vi "MultiPAS-IV.vi"() -> ()   [LabVIEW 2011]
uses:
  Desktop/__fcncfs4.franklin.uga.edu_CHEM/Groups/Smith_G/Photoacoutic Spectroscopy/PAS-CRD/Get Tau/Analysis/analys_meth.ctl
  <vilib>/Analysis/4window.llb/windowTd.ctl
  sub/QMH/QMH Add Message to Queue (Single Element).vi
  sub/QMH/QMH Add Message to Queue (Array).vi
  <vilib>/measure/maspectr.llb/FFT Spectrum (Mag-Phase) for 1 Chan.vi
  sub/fftGetMags_IV.vi
  sub/rollingAverage_IV.vi
  sub/micUnbundle_IV.vi
  sub/laserDiagnose_IV.vi
  <vilib>/Instr/_visa.llb/VISA Configure Serial Port (Instr).vi
  sub/lasersSetFrequencies_IV.vi
  sub/absCalcPlot_IV.vi
  sub/pdNormalize_IV.vi
  <vilib>/measure/NI_MAPro.lvlib
  <vilib>/Analysis/NI_AALPro.lvlib
panel:
  out "Channel A":cluster{i32, sgl, "Data (mV)":dbl[]}(graph)
  out "tau":dbl(graph)
  in  "785 Emission":bool
  in  "785 Power (mW)":dbl(slide)=100.0 min=0.0 max=100.0 step=1.0 scale=0.0..100.0
  out "PAS Save":bool caption="Overtemp"
  in  "Data 2":i32[][](array[numeric])=[[-16374, -7248, 2543, 12030, 20279, 26487, 30037, 30583, 28073, 22744, 15131, 5976, -3818, -13288, -21504, -27663, -31155, -31636, -29064, -23686, -16036, -6862, 2936, 12388, 20571, 26684, 30122, 30546, 27911, 22483, 14793, 5595, -4207, -13644, -21795, -27855, -31232, -31591, -28898, -23423, -15695, -6476, 3323, 12743, 20858, 26873, 30194, 30492, 27744, 22213, 14447, 5207, -4597, -14002, -22082, -28044, -31304, -31540, -28731, -23149, -15348, -6093, 3713, 13101, 21145, 27063, 30265, 30442, 27576, 21943, 14103, 4822, -4984, -14354, -22365, -28230, -31373, -31485, -28556, -22876, -14998, -5702, 4104, 13452, 21428, 27245, 30335, 30388, 27400, 21669, 13754, 4435, -5375, -14705, -22643, -28407, -31436, -31426, -28378, -22598, -14648, -5314, 4497, 13803, 21706, 27423, 30394, 30325, 27221, 21390, 13402, 4045, -5763, -15056, -22921, -28586, -31496, -31361, -28198, -22319, -14297, -4924, 4879, 14151, 21982, 27597, 30451, 30257, 27038, 21107, 13050, 3658, -6149, -15402, -23193, -28754, -31546, -31290, -28010, -22033, -13944, -4536, 5266, 14498, 22252, 27767, 30500, 30184, 26849, 20821, 12696, 3267, -6535, -15748, -23462, -28924, -31596, -31216, -27821, -21748, -13587, -4147, 5653, 14838, 22519, 27930, 30549, 30110, 26658, 20535, 12337, 2878, -6919, -16089, -23727, -29087, -31641, -31137, -27627, -21457, -13229, -3753, 6038, 15181, 22786, 28093, 30591, 30031, 26461, 20243, 11979, 2485, -7303, -16428, -23991, -29244, -31678, -31053, -27426, -21159, -12867, -3360, 6424, 15524, 23043, 28252, 30633, 29946, 26262, 19946, 11617, 2096, -7686, -16764, -24246, -29398, -31712, -30964, -27224, -20862, -12503, -2971, 6803, 15859, 23301, 28401, 30661, 29852, 26058, 19648, 11254, 1703, -8069, -17099, -24500, -29547, -31741, -30870, -27018, -20562, -12138, -2575, 7188, 16192, 23556, 28549, 30689, 29756, 25848, 19348, 10891, 1312, -8448, -17430, -24753, -29691, -31765, -30773, -26806, -20259, -11775, -2186, 7566, 16521, 23801, 28690, 30709, 29656, 25634, 19038, 10523, 919, -8831, -17762, -24997, -29833, -31788, -30672, -26593, -19955, -11409, -1792, 7944, 16850, 24047, 28830, 30724, 29548, 25416, 18729, 10152, 523, -9212, -18092, -25245, -29969, -31805, -30566, -26375, -19647, -11041, -1403, 8319, 17173, 24287, 28963, 30734, 29436, 25192, 18418, 9781, 130, -9587, -18413, -25481, -30101, -31814, -30449, -26150, -19332, -10666, -1007, 8697, 17497, 24524, 29090, 30745, 29325, 24968, 18105, 9408, -263, -9962, -18735, -25718, -30228, -31820, -30334, -25921, -19016, -10296, -618, 9072, 17814, 24756, 29213, 30746, 29202, 24738, 17787, 9036, -657, -10338, -19058, -25951, -30350, -31818, -30214, -25690, -18699, -9922, -224, 9442, 18128, 24984, 29330, 30738, 29078, 24502, 17466, 8658, -1050, -10710, -19371, -26178, -30467, -31814, -30088, -25458, -18382, -9550, 167, 9812, 18440, 25206, 29443, 30732, 28947, 24264, 17143, 8281, -1445, -11083, -19685, -26404, -30581, -31807, -29959, -25221, -18059, -9175, 556, 10178, 18750, 25426, 29548, 30718, 28809, 24018, 16812, 7901, -1842, -11457, -19996, -26624, -30690, -31795, -29824, -24980, -17733, -8799, 950, 10549, 19058, 25643, 29655, 30700, 28673, 23773, 16484, 7523, -2235, -11824, -20304, -26840, -30793, -31772, -29682, -24731, -17402, -8415, 1341, 10916, 19363, 25856, 29755, 30677, 28528, 23522, 16151, 7141, -2626, -12191, -20607, -27051, -30891, -31746, -29536, -24481, -17070, -8035, 1733, 11280, 19664, 26064, 29851, 30648, 28381, 23272, 15818, 6762, -3019, -12555, -20906, -27258, -30984, -31717, -29391, -24226, -16736, -7655, 2128, 11641, 19962, 26270, 29940, 30615, 28229, 23013, 15483, 6376, -3409, -12914, -21204, -27459, -31071, -31684, -29236, -23967, -16398, -7271, 2515, 12005, 20258, 26468, 30024, 30577, 28072, 22753, 15143, 5990, -3802, -13276, -21497, -27660, -31157, -31643, -29076, -23707, -16058, -6886, 2908, 12363, 20550, 26666, 30107, 30536, 27914, 22489, 14805, 5607, -4192, -13633, -21787, -27849, -31230, -31597, -28911, -23438, -15716, -6501, 3298, 12719, 20839, 26858, 30182, 30488, 27744, 22223, 14459, 5225, -4579, -13988, -22071, -28040, -31304, -31549, -28743, -23167, -15368, -6113, 3693, 13076, 21126, 27047, 30255, 30438, 27576, 21950, 14113, 4837, -4971, -14340, -22354, -28224, -31375, -31494, -28570, -22895, -15022, -5725, 4080, 13430, 21408, 27230, 30324, 30384, 27402, 21676, 13766, 4449, -5360, -14694, -22636, -28409, -31440, -31436, -28397, -22617, -14674, -5338, 4467, 13781, 21686, 27408, 30385, 30320, 27224, 21398, 13418, 4062, -5748, -15044, -22913, -28584, -31498, -31368, -28212, -22339, -14321, -4948, 4856, 14131, 21963, 27583, 30440, 30254, 27042, 21118, 13062, 3669, -6137, -15390, -23183, -28751, -31551, -31297, -28024, -22049, -13962, -4556, 5245, 14476, 22235, 27754, 30497, 30186, 26857, 20834, 12710, 3283, -6519, -15733, -23453, -28921, -31600, -31226, -27837, -21765, -13610, -4168, 5628, 14820, 22502, 27918, 30540, 30109, 26664, 20544, 12354, 2891, -6906, -16074, -23719, -29085, -31646, -31148, -27642, -21475, -13251, -3777, 6014, 15160, 22765, 28078, 30583, 30027, 26468, 20251, 11994, 2501, -7292, -16415, -23980, -29242, -31682, -31064, -27443, -21181, -12892, -3386, 6397, 15501, 23026, 28238, 30624, 29944, 26269, 19959, 11633, 2110, -7673, -16753, -24239, -29395, -31719, -30974, -27239, -20882, -12528, -2993, 6782, 15835, 23285, 28390, 30651, 29852, 26063, 19660, 11271, 1720, -8053, -17087, -24493, -29546, -31746, -30880, -27031, -20583, -12163, -2599, 7166, 16173, 23538, 28538, 30684, 29758, 25853, 19356, 10906, 1327, -8433, -17416, -24743, -29688, -31769, -30782, -26821, -20280, -11797, -2208, 7543, 16501, 23786, 28680, 30704, 29656, 25642, 19053, 10540, 936, -8814, -17747, -24989, -29827, -31787, -30678, -26606, -19973, -11430, -1817, 7923, 16829, 24031, 28819, 30721, 29552, 25424, 18746, 10174, 543, -9191, -18072, -25231, -29962, -31802, -30567, -26384, -19660, -11057, -1422, 8302, 17159, 24274, 28952, 30738, 29443, 25205, 18435, 9801, 150, -9568, -18401, -25472, -30095, -31811, -30457, -26163, -19349, -10687, -1031, 8679, 17481, 24511, 29082, 30742, 29327, 24979, 18121, 9431, -241, -9943, -18717, -25707, -30221, -31815, -30337, -25930, -19029, -10312, -631, 9058, 17802, 24745, 29207, 30746, 29209, 24750, 17805, 9057, -634, -10316, -19037, -25937, -30340, -31814, -30217, -25700, -18713, -9939, -240, 9429, 18117, 24976, 29328, 30740, 29088, 24519, 17486, 8682, -1027, -10688, -19352, -26164, -30458, -31810, -30091, -25465, -18390, -9561, 154, 9800, 18433, 25201, 29442, 30735, 28959, 24282, 17165, 8308, -1420, -11063, -19665, -26386, -30570, -31801, -29961, -25227, -18068, -9185, 547, 10171, 18745, 25424, 29552, 30726, 28825, 24038, 16835, 7925, -1815, -11429, -19974, -26608, -30681, -31789, -29826, -24984, -17741, -8807, 938, 10536, 19047, 25636, 29657, 30708, 28685, 23794, 16510, 7550, -2205, -11798, -20280, -26821, -30782, -31766, -29684, -24737, -17411, -8429, 1331, 10906, 19356, 25851, 29758, 30684, 28544, 23546, 16178, 7169, -2598, -12162, -20582, -27035, -30879, -31744, -29540, -24485, -17080, -8048, 1721, 11267, 19655, 26061, 29852, 30654, 28395, 23291, 15843, 6786, -2993, -12527, -20884, -27240, -30974, -31713, -29390, -24230, -16744, -7662, 2115, 11635, 19957, 26268, 29945, 30624, 28246, 23035, 15509, 6406, -3382, -12889, -21180, -27444, -31061, -31677, -29236, -23975, -16408, -7284], [-19329, -1252, 17344, 29341, 30145, 19451, 1353, -17227, -29174, -29920, -19175, -1056, 17506, 29408, 30095, 19300, 1159, -17387, -29238, -29860, -19019, -860, 17671, 29475, 30037, 19143, 960, -17553, -29307, -29809, -18866, -664, 17832, 29545, 29987, 18991, 771, -17707, -29365, -29749, -18707, -466, 17992, 29605, 29926, 18832, 570, -17873, -29434, -29694, -18556, -272, 18151, 29670, 29869, 18676, 375, -18031, -29495, -29633, -18395, -75, 18310, 29729, 29809, 18516, 175, -18194, -29561, -29579, -18238, 120, 18469, 29792, 29750, 18362, -17, -18347, -29617, -29515, -18076, 316, 18629, 29848, 29682, 18197, -218, -18510, -29679, -29456, -17921, 513, 18787, 29910, 29626, 18042, -408, -18664, -29734, -29388, -17757, 709, 18941, 29965, 29560, 17875, -609, -18823, -29791, -29326, -17600, 904, 19095, 30023, 29495, 17717, -802, -18975, -29845, -29260, -17434, 1099, 19251, 30075, 29425, 17551, -1001, -19131, -29901, -29194, -17277, 1296, 19408, 30130, 29359, 17393, -1193, -19284, -29953, -29124, -17112, 1491, 19560, 30184, 29290, 17225, -1392, -19440, -30008, -29056, -16949, 1686, 19713, 30237, 29226, 17069, -1581, -19587, -30054, -28982, -16781, 1883, 19866, 30287, 29151, 16898, -1781, -19742, -30107, -28913, -16616, 2079, 20018, 30337, 29082, 16737, -1973, -19888, -30152, -28838, -16449, 2275, 20167, 30383, 29006, 16564, -2174, -20041, -30200, -28765, -16282, 2471, 20321, 30430, 28934, 16403, -2364, -20187, -30243, -28688, -16113, 2669, 20465, 30470, 28853, 16230, -2568, -20341, -30294, -28618, -15953, 2860, 20615, 30519, 28783, 16070, -2755, -20486, -30335, -28537, -15779, 3057, 20760, 30560, 28700, 15892, -2956, -20637, -30378, -28461, -15613, 3252, 20909, 30605, 28628, 15730, -3145, -20777, -30418, -28377, -15440, 3446, 21054, 30645, 28543, 15557, -3345, -20927, -30460, -28299, -15271, 3643, 21199, 30686, 28465, 15391, -3534, -21066, -30495, -28215, -15100, 3839, 21345, 30722, 28380, 15214, -3734, -21213, -30534, -28134, -14928, 4032, 21487, 30760, 28300, 15044, -3926, -21355, -30570, -28052, -14757, 4225, 21627, 30792, 28209, 14870, -4123, -21501, -30607, -27968, -14586, 4419, 21768, 30832, 28129, 14702, -4314, -21637, -30639, -27880, -14413, 4612, 21907, 30859, 28040, 14521, -4515, -21780, -30675, -27796, -14241, 4804, 22048, 30895, 27953, 14352, -4702, -21919, -30705, -27707, -14064, 4999, 22187, 30922, 27859, 14172, -4900, -22060, -30739, -27620, -13892, 5193, 22326, 30954, 27773, 14003, -5090, -22194, -30765, -27524, -13712, 5386, 22462, 30981, 27679, 13823, -5285, -22333, -30794, -27436, -13538, 5580, 22600, 31013, 27591, 13650, -5476, -22466, -30820, -27343, -13363, 5770, 22732, 31033, 27491, 13468, -5673, -22605, -30848, -27251, -13187, 5964, 22870, 31060, 27401, 13292, -5863, -22736, -30870, -27155, -13010, 6156, 23000, 31079, 27299, 13111, -6058, -22873, -30895, -27060, -12833, 6347, 23134, 31104, 27208, 12936, -6248, -23004, -30918, -26965, -12652, 6536, 23260, 31120, 27106, 12753, -6444, -23136, -30939, -26865, -12472, 6729, 23395, 31148, 27011, 12578, -6634, -23266, -30959, -26766, -12296, 6919, 23523, 31161, 26907, 12392, -6830, -23402, -30982, -26665, -12115, 7109, 23652, 31180, 26809, 12213, -7016, -23524, -30992, -26564, -11932, 7301, 23777, 31195, 26704, 12032, -7210, -23655, -31011, -26464, -11755, 7492, 23907, 31211, 26605, 11855, -7395, -23778, -31024, -26358, -11573, 7680, 24031, 31218, 26494, 11665, -7592, -23908, -31039, -26258, -11392, 7871, 24158, 31237, 26394, 11491, -7775, -24031, -31050, -26153, -11210, 8063, 24281, 31247, 26285, 11302, -7972, -24159, -31062, -26046, -11027, 8250, 24407, 31258, 26180, 11124, -8157, -24276, -31067, -25937, -10841, 8438, 24526, 31265, 26071, 10936, -8347, -24401, -31078, -25829, -10659, 8630, 24649, 31275, 25965, 10755, -8533, -24522, -31087, -25721, -10474, 8816, 24770, 31280, 25853, 10566, -8726, -24641, -31091, -25608, -10290, 9003, 24891, 31287, 25746, 10386, -8910, -24756, -31095, -25498, -10105, 9192, 25008, 31287, 25627, 10196, -9102, -24881, -31101, -25386, -9919, 9381, 25127, 31296, 25521, 10019, -9284, -24994, -31099, -25268, -9732, 9570, 25243, 31293, 25403, 9826, -9476, -25113, -31105, -25157, -9544, 9756, 25359, 31298, 25291, 9645, -9655, -25225, -31099, -25040, -9359, 9942, 25473, 31291, 25167, 9453, -9847, -25341, -31102, -24926, -9173, 10124, 25586, 31294, 25057, 9269, -10029, -25450, -31095, -24809, -8986, 10310, 25696, 31284, 24931, 9078, -10218, -25564, -31094, -24688, -8798, 10497, 25812, 31287, 24819, 8896, -10399, -25673, -31085, -24567, -8608, 10682, 25922, 31278, 24698, 8703, -10587, -25785, -31080, -24448, -8422, 10866, 26033, 31274, 24582, 8522, -10765, -25890, -31067, -24321, -8230, 11050, 26140, 31263, 24455, 8325, -10952, -26001, -31064, -24201, -8040, 11234, 26248, 31255, 24338, 8142, -11132, -26106, -31054, -24079, -7852, 11417, 26353, 31243, 24207, 7948, -11316, -26217, -31041, -23952, -7662, 11601, 26464, 31236, 24089, 7763, -11494, -26315, -31025, -23829, -7471, 11782, 26562, 31217, 23957, 7567, -11682, -26422, -31014, -23702, -7282, 11962, 26667, 31205, 23834, 7383, -11859, -26521, -30998, -23575, -7092, 12144, 26770, 31187, 23704, 7186, -12043, -26626, -30981, -23444, -6900, 12328, 26875, 31176, 23582, 7003, -12218, -26724, -30962, -23316, -6709, 12505, 26971, 31154, 23446, 6805, -12401, -26825, -30946, -23189, -6517, 12687, 27073, 31139, 23322, 6620, -12576, -26919, -30922, -23054, -6323, 12867, 27170, 31114, 23185, 6422, -12760, -27022, -30904, -22923, -6132, 13047, 27272, 31096, 23060, 6237, -12934, -27114, -30879, -22790, -5940, 13222, 27362, 31068, 22921, 6041, -13116, -27212, -30855, -22657, -5748, 13401, 27461, 31048, 22790, 5853, -13289, -27302, -30828, -22522, -5555, 13577, 27549, 31019, 22652, 5652, -13472, -27398, -30806, -22388, -5362, 13753, 27645, 30995, 22521, 5463, -13642, -27487, -30776, -22248, -5169, 13928, 27733, 30963, 22376, 5266, -13823, -27584, -30750, -22113, -4975, 14106, 27828, 30937, 22246, 5082, -13992, -27669, -30717, -21974, -4782, 14280, 27914, 30902, 22101, 4880, -14174, -27760, -30689, -21837, -4588, 14454, 28006, 30875, 21965, 4692, -14340, -27843, -30653, -21693, -4391, 14631, 28092, 30840, 21822, 4494, -14519, -27934, -30620, -21552, -4198, 14805, 28179, 30808, 21688, 4308, -14687, -28015, -30582, -21410, -4004, 14975, 28262, 30770, 21540, 4106, -14861, -28103, -30548, -21268, -3808, 15149, 28349, 30739, 21402, 3916, -15032, -28183, -30512, -21124, -3614, 15319, 28430, 30697, 21255, 3715, -15205, -28267, -30475, -20982, -3421, 15490, 28513, 30664, 21116, 3524, -15376, -28348, -30435, -20837, -3225, 15660, 28592, 30617, 20962, 3327, -15550, -28432, -30397, -20695, -3032, 15829, 28673, 30581, 20820, 3134, -15711, -28506, -30353, -20546, -2837, 15994, 28746, 30530, 20669, 2933, -15887, -28585, -30311, -20400, -2641, 16167, 28828, 30496, 20528, 2745, -16052, -28660, -30264, -20248, -2445, 16335, 28901, 30445, 20376, 2544, -16221, -28737, -30219, -20102, -2250, 16505, 28983, 30406, 20231, 2357, -16381, -28808, -30171, -19950, -2053, 16670, 29053, 30355, 20075, 2154, -16552, -28883, -30127, -19803, -1859, 16835, 29128, 30308, 19930, 1965, -16714, -28952, -30073, -19650, -1663, 17001, 29192, 30255, 19772, 1764, -16881, -29028, -30026, -19496, -1467, 17165, 29268, 30208, 19626, 1572, -17043, -29095, -29977, -19346]]
  out "Filtering":bool caption="Time has Elapsed"
  in  "Switch Filter":bool
  in  "Auto Filter":bool
  out "Elapsed Time (min)":dbl caption="Elapsed Time (s)" format="%#.1g"
  in  "Filter Length (min)":dbl=6.0 caption="Time Target (s)"
  in  "Sample Length (min)":dbl=24.0 caption="Time Target (s)" format="%#.1f"
  out "Time has Elapsed":bool
  in  "Time Target (s)":dbl=1.0
  in  "sweep":bool
  in  "All Emit":bool
  in  "Alignment Mode":bool
  in  "662 Emission":bool
  in  "662 Power (mW)":dbl(slide)=100.0 min=0.0 max=100.0 step=1.0 scale=0.0..100.0
  in  "532 Emission":bool
  in  "532 Power (mW)":dbl(slide)=80.0 min=0.0 max=80.0 step=1.0 scale=0.0..80.0
  in  "406 Power (mW)":dbl(slide)=100.0 min=0.0 max=100.0 step=1.0 scale=0.0..100.0
  in  "406 Emission":bool
  out "Overtemp":bool
  in  "Tab Control":T1(tab)=enum."Oscilloscope"
  out "crd":path
  in  "785 Port":refnum<visa-resource-name>="COM81"
  in  "785 PD Cal":dbl=0.039
  out "Error Console":T2
  out "pd":path caption="Photodiode File Path"
  out "mic":path caption="Microphone File Path"
  out "processed":path caption="Processed Data File Path"
  out "sweeps":path caption="Frequency Sweeps File Path"
  out "Laser Temperatures":T3(graph)
  in  "pd id":u32=1
  in  "mic id":u32
  in  "mic cal, scu":dbl=5.41531278804282e-05 format="%#_3e"
  in  "mic cal, scu":dbl=5.59307241877627e-05 format="%#_3e"
  in  "406 Port":refnum<visa-resource-name>="COM80"
  in  "532 Port":refnum<visa-resource-name>="COM79"
  in  "662 Port":refnum<visa-resource-name>="COM62"
  in  "Teensy Port":refnum<visa-resource-name>="COM78"
  in  "Save Data":bool
  in  "405 PD Cal 3":dbl=0.052
  in  "532 PD Cal 3":dbl=0.035
  in  "660 PD Cal 3":dbl=0.038
  in  "Channel A Settings":T4={"Enabled"=TRUE, "Coupling"=0, "Range"=1, "Analogue Offset"=0.0} {"Range" items=["20 mV"=1, "50 mV"=2, "100 mV"=3, "200 mV"=4, "500 mV"=5, "1 V"=6, "2 V"=7, "5 V"=8, "10 V"=9, "20 V"=10]; "Coupling" items=["AC", "DC"]}
  in  "Trigger Settings":T5={"Trigger Enabled"=TRUE, "Trigger Source"=enum."Channel B", "Trigger Threshold (V)"=1.0, "Trigger Direction"=3, "Trigger Delay (samples)"=0, "Auto Trigger Time (ms)"=1000} {"Trigger Direction" items=["Rising"=2, "Falling"=3]}
  in  "Acquisition Settings":T6={"Pre-trigger Samples"=0, "Post-trigger Samples"=10000, "Timebase"=1, "Down Sample Ratio"=10, "Oversample"=1, "Number of Captures"=100, "Down-Sample Mode"=4} {"Down-Sample Mode" items=["None"=0, "Aggregate"=1, "Decimate"=2, "Average"=4]; "Down Sample Ratio" min=1 step=1}
  in  "Channel B Settings":T4={"Enabled"=TRUE, "Coupling"=1, "Range"=8, "Analogue Offset"=0.0} {"Range" items=["20 mV"=1, "50 mV"=2, "100 mV"=3, "200 mV"=4, "500 mV"=5, "1 V"=6, "2 V"=7, "5 V"=8, "10 V"=9, "20 V"=10]; "Coupling" items=["AC", "DC"]}
  in  "785 F (Hz)":i32=1371
  out "freqscan":cluster{i32[], "Best Gaussian Fit":dbl[]}[](graph) caption="Frequency Sweep"
  out "sweep progress":dbl(slide) scale=0.0..1.0
  in  "Autosweep?":bool=TRUE
  in  "set freqs":bool
  out "Calculated Resonance (Hz)":dbl=1370.0
  in  "Data Start Frequency (Hz)":i32=1355
  in  "Data End Frequency (Hz)":i32=1405
  in  "423 F (Hz)":i32=1367
  in  "532 F (Hz)":i32=1373
  in  "662 F (Hz)":i32=1369
  in  "Chart Rolling Average":i32=64
  out "pdwave":waveform(i32)(graph) caption="Photodiode Waveform"
  out "pd ts":cluster{dbl, dbl, dbl, dbl}(graph)
  out "pdfft":cluster{"f0":dbl, "df":dbl, "magnitude":dbl[]}(graph) caption="Photodiode FFT"
  in  "rollavg":i32=16 caption="Dispaly Averaging\n(Transfers to Abs!)"
  out "mic ts":T7(graph)
  out "micfft":cluster{"f0":dbl, "df":dbl, "magnitude":dbl[]}(graph) caption="Photodiode FFT"
  out "micwave":waveform(i32)(graph) caption="Photodiode Waveform"
  out "abs/ext":cluster{dbl, dbl, dbl, dbl, "crd":dbl}(graph)
  in  "getbkg":bool
  out "AAE":dbl(graph)
  in  "Bkg Values (mV)":cluster{dbl, dbl, dbl, dbl}
  out "Absorption Spectrum":cluster{dbl[], "Best Power Fit":dbl[]}[](graph)
  in  "cellcal":dbl=100000.0 caption="Cell Calibration Coefficient (mV/mW)"
  in  "tau0":dbl
  out "Status":string
  in  "Exit":bool
  in  "State Variables":cluster{"CurrentFile":path}
  # "MultiPAS-IV | AeroSmith Labs (2017)"
  # "Laser Control"
  # "Filter Control"
  # "Communications"
  # "Sound Card Parameters"
  # "File paths are populated automatically at <...\\My Documents\\MultiPAS Data\\>.  To save in another location, turn on \"Save Data\" and follow the prompts to choose an alternate working directory."
  # "Photodiode Calibration"
  # "Ringdown Time (us):"
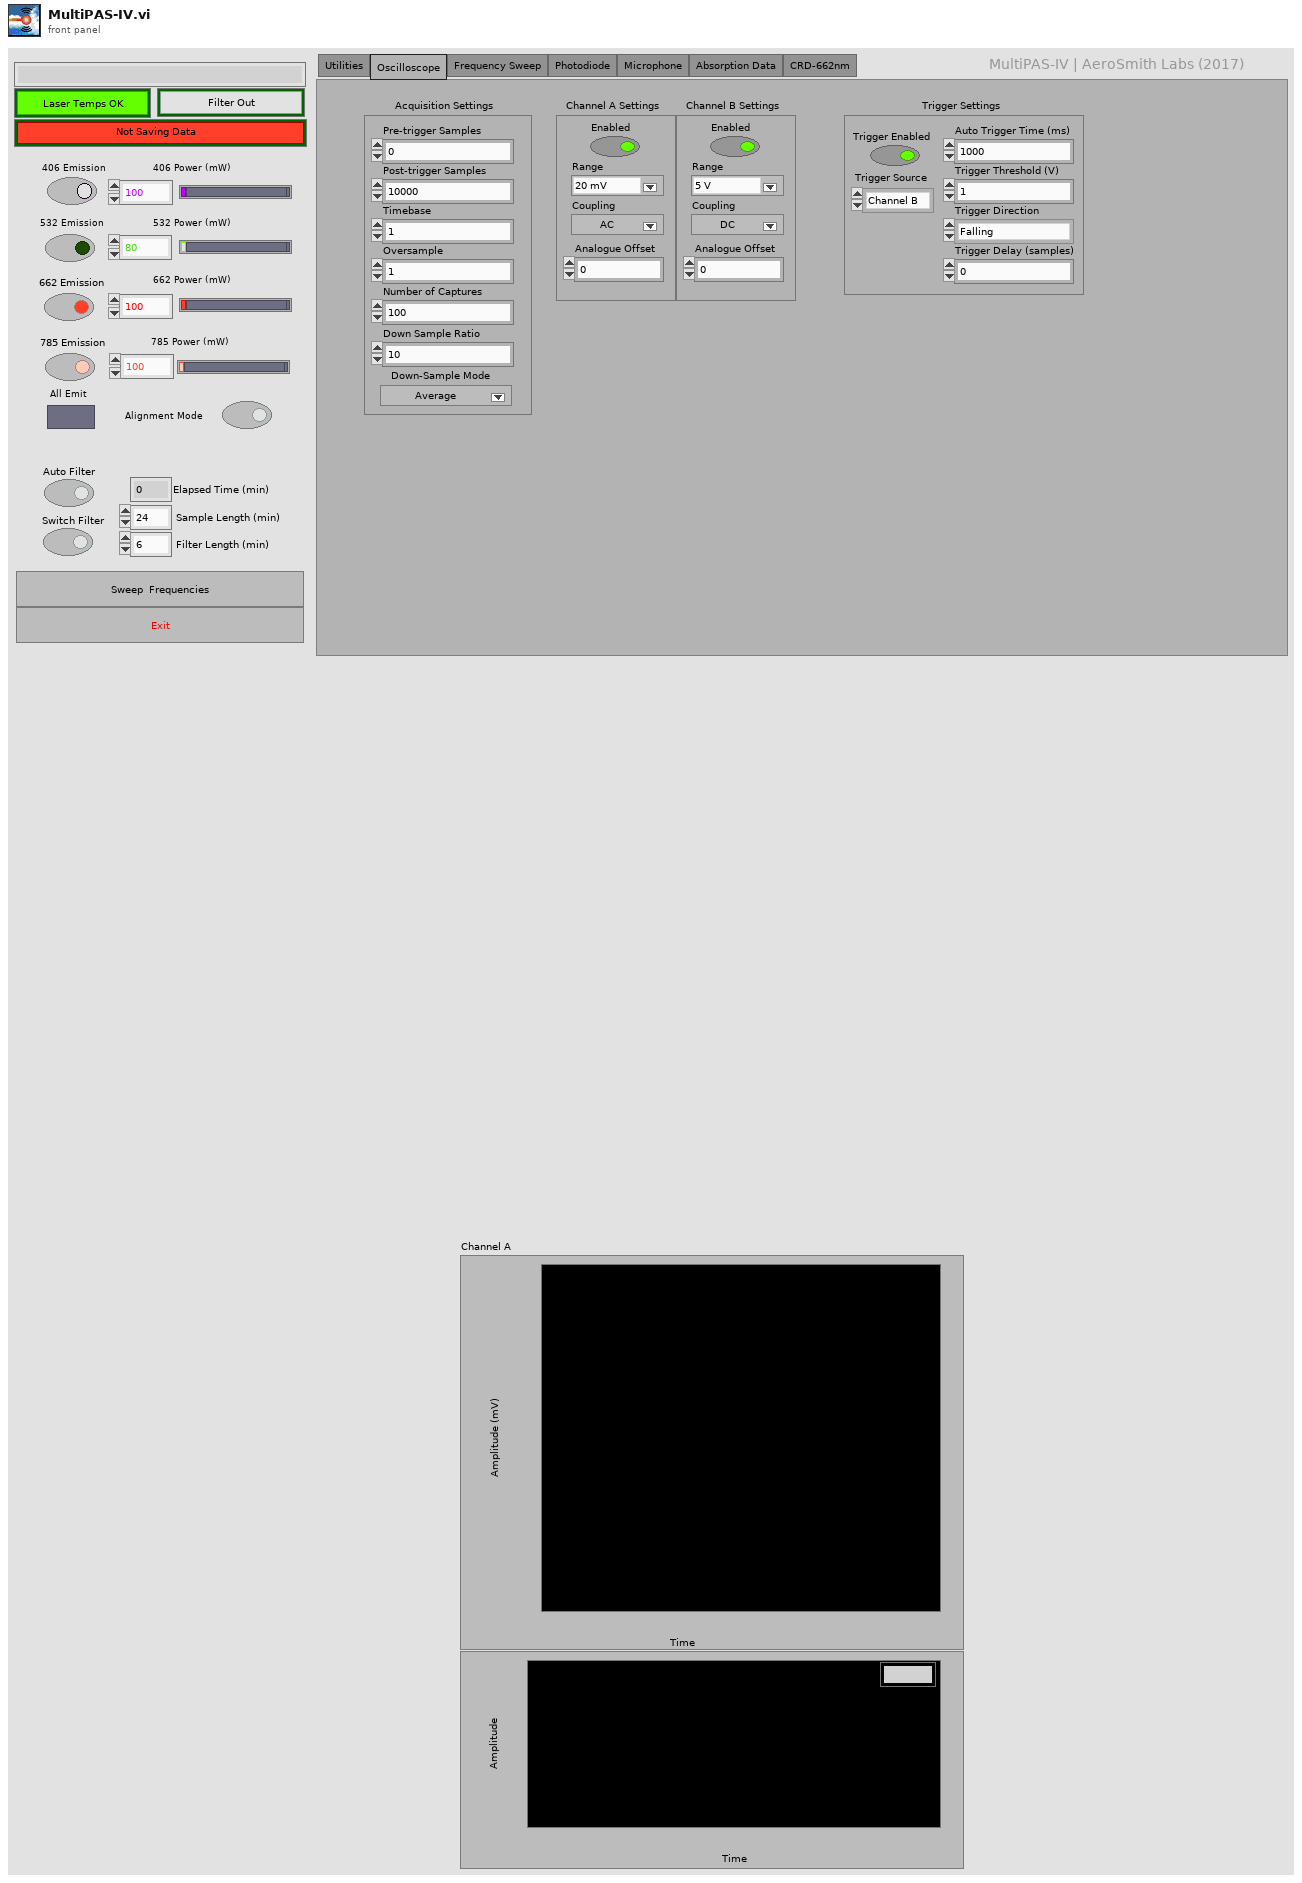
[diagram p1: front panel]
types:
  T1 = enum32{"Utilities", "Oscilloscope", "Frequency Sweep", "Photodiode", "Microphone", "Absorption Data", "CRD-662nm"}
  T2 = cluster{"status":bool, "code":i32, "Message":string}
  T3 = cluster{"Temp (C)":dbl, "Temp (C)":dbl, "Temp (C)":dbl, "Temp (C)":dbl}
  T4 = cluster{"Enabled":bool, "Coupling":i16, "Range":u16, "Analogue Offset":sgl}
  T5 = cluster{"Trigger Enabled":bool, "Trigger Source":enum16{"Channel A", "Channel B", "Channel C", "Channel D", "Ext."}, "Trigger Threshold (V)":dbl, "Trigger Direction":u16, "Trigger Delay (samples)":u32, "Auto Trigger Time (ms)":i16}
  T6 = cluster{"Pre-trigger Samples":u32, "Post-trigger Samples":u32, "Timebase":u32, "Down Sample Ratio":u32, "Oversample":i16, "Number of Captures":u32, "Down-Sample Mode":i32}
  T7 = cluster{"422 Mean":dbl, "532 Mean":dbl, "660 Mean":dbl, "785 Mean":dbl}
  T8 = cluster{"# buffers":i32, "Buffer size":i32, "unit (ms)":enum16{"time (ms)", "Samples"}}
  T9 = typedef "SoundHandle.ctl" = cluster{"DeviceID":u16, "Samples/buf":u32, "Sampl rate":u32, "Bits/sample":u16, "Channels":u8, "Opened":bool}
  T10 = cluster{"405 Mean":dbl, "532 Mean":dbl, "660 Mean":dbl, "660 Mean 2":dbl}
  T11 = typedef "NI_AALPro.lvlib/windowTd.ctl" = u32
  T12 = cluster{"785 New Array":dbl[], "785 Mean":dbl, "785 SD":dbl}
  T13 = cluster{"660 New Array":dbl[], "660 Mean":dbl, "660 SD":dbl}
  T14 = cluster{"532 New Array":dbl[], "532 Mean":dbl, "532 SD":dbl}
  T15 = cluster{"405 New Array":dbl[], "405 Mean":dbl, "405 SD":dbl}
  T16 = typedef "analys_meth.ctl" = enum16{"DFT-1", "DFT-5", "LRS"}
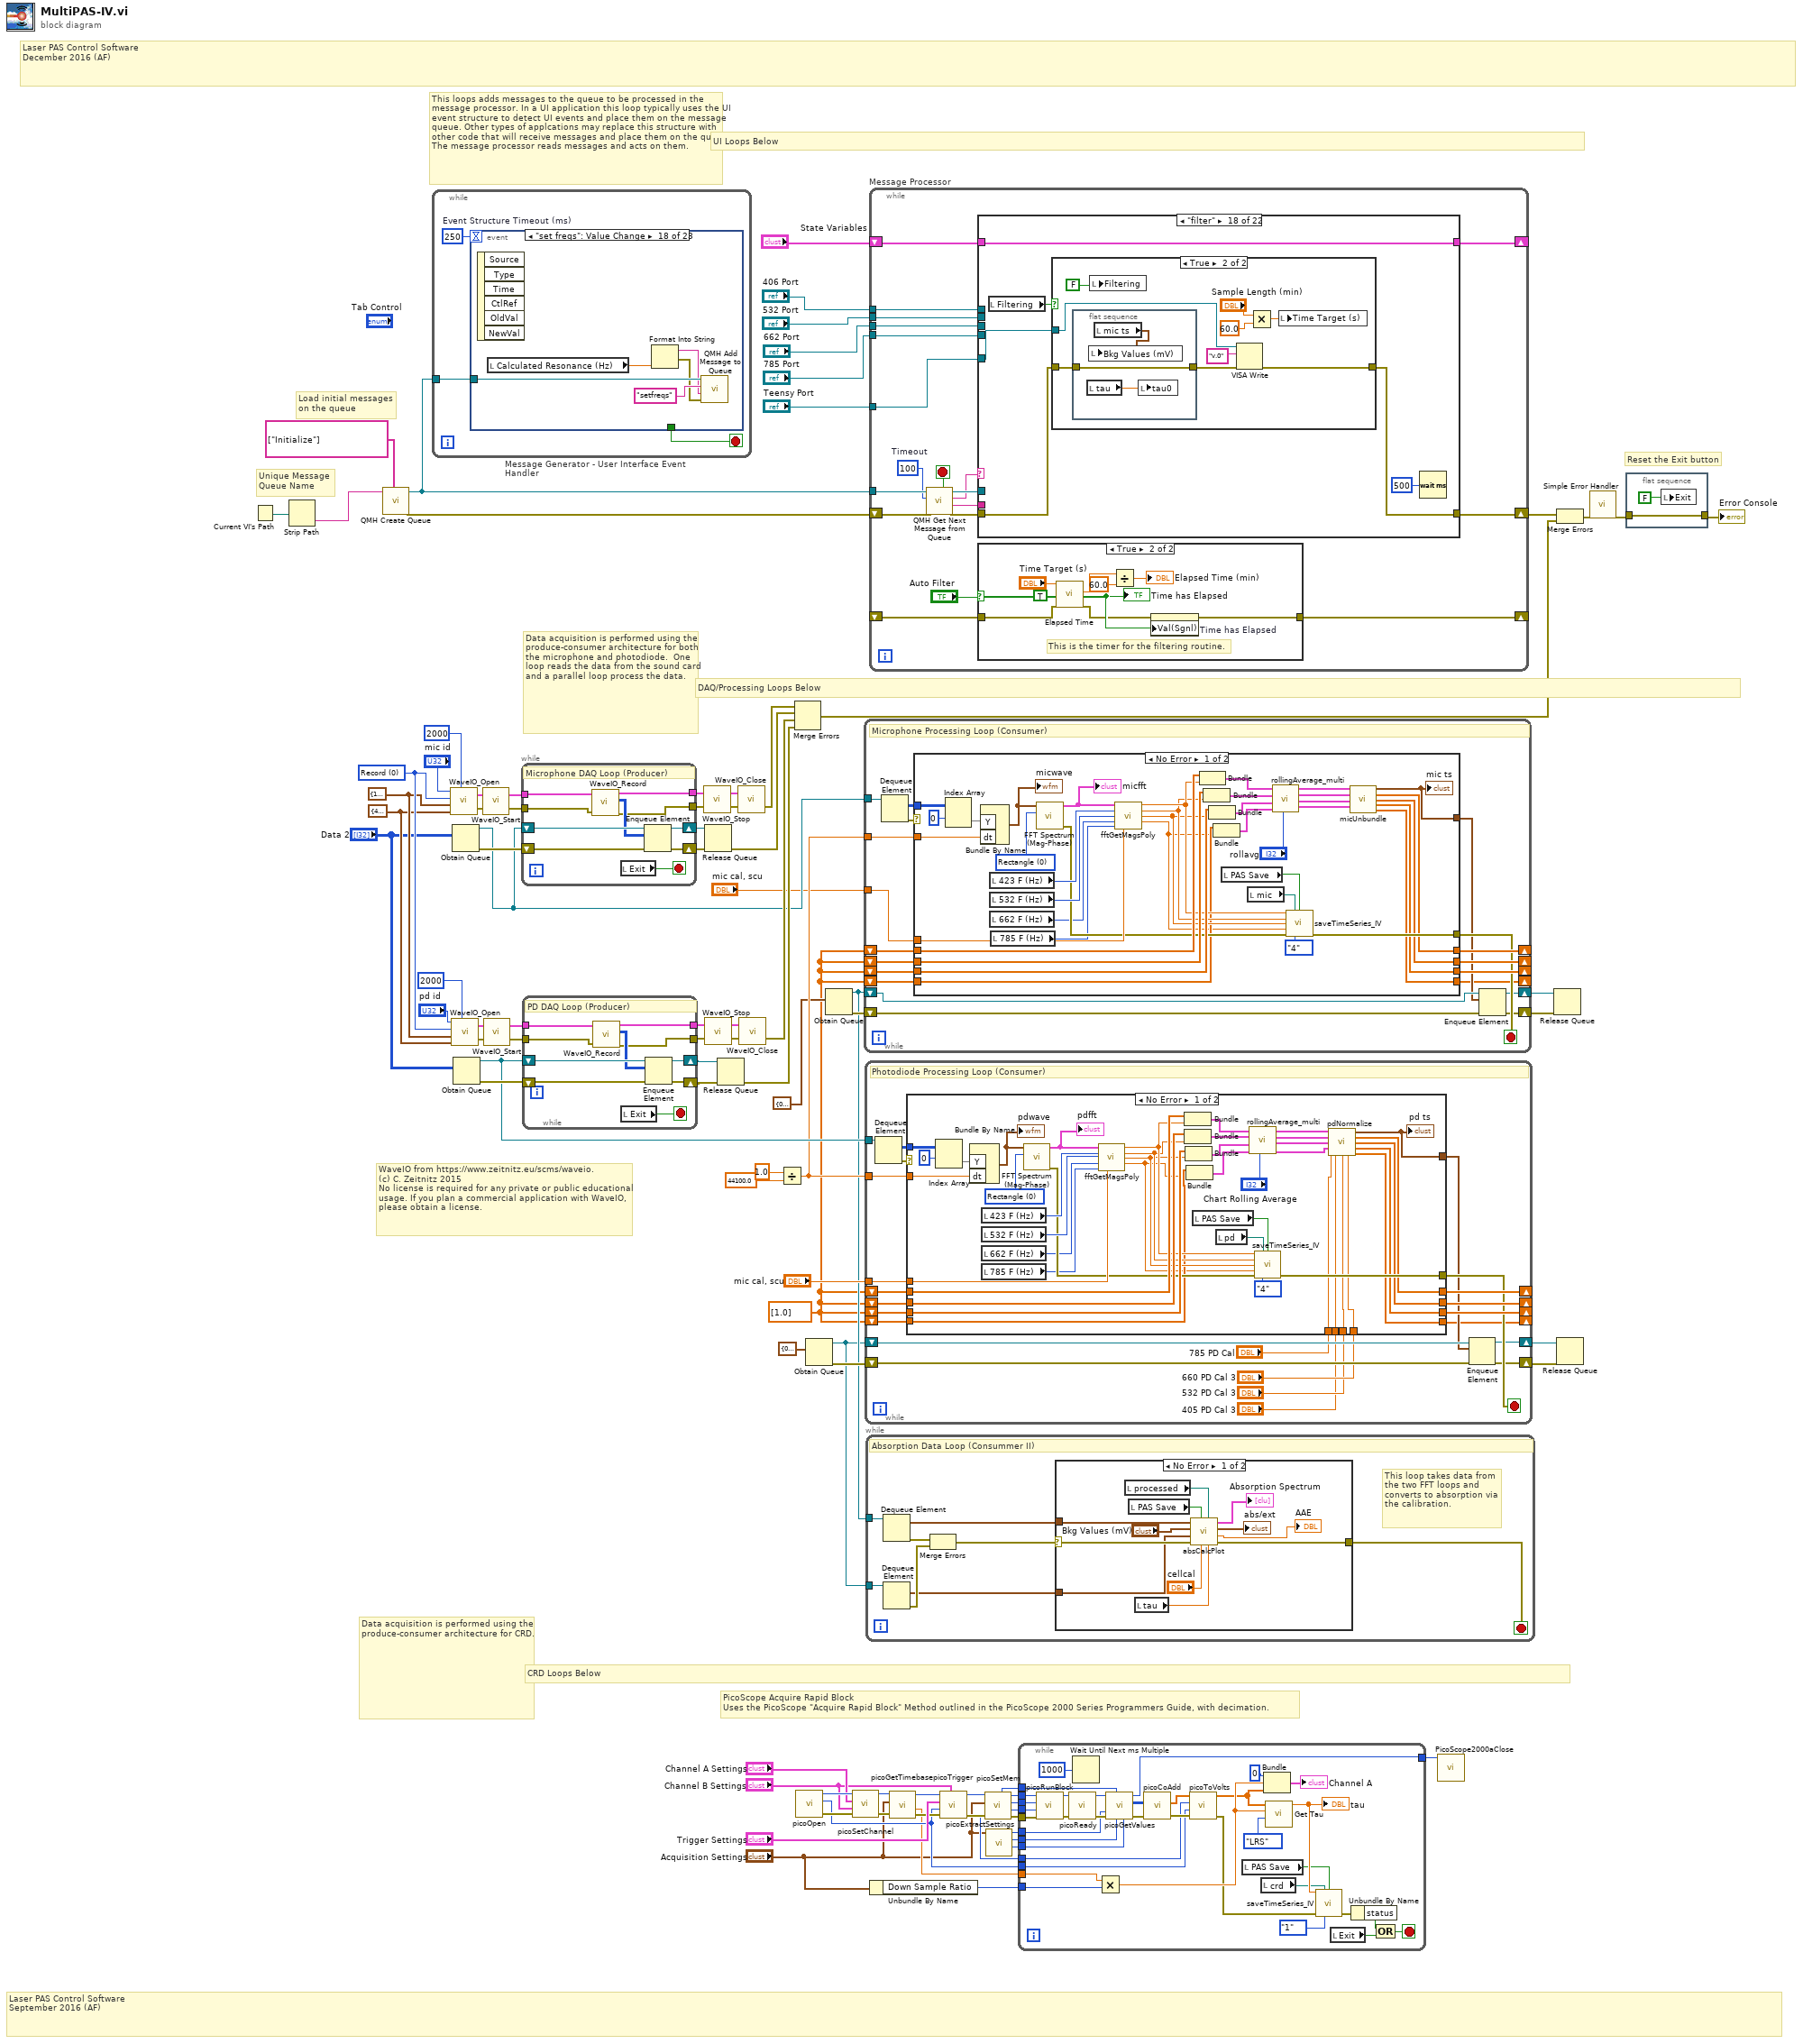
[diagram p0: block diagram]
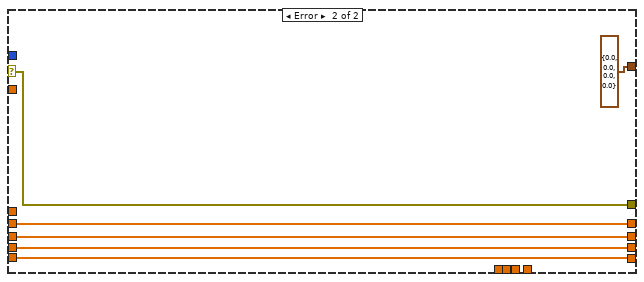
[diagram p3: hidden frame]
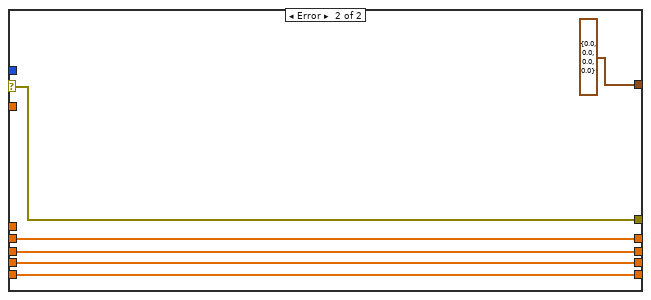
[diagram p4: hidden frame]
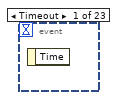
[diagram p5: hidden frame]
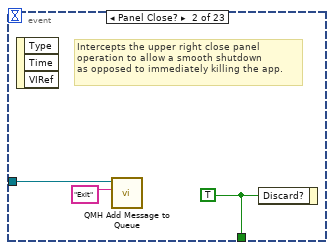
[diagram p6: hidden frame]
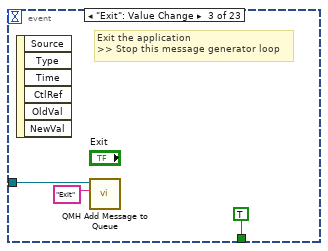
[diagram p7: hidden frame]
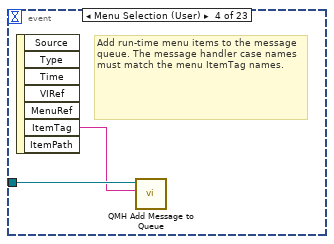
[diagram p8: hidden frame]
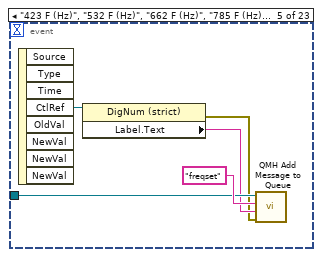
[diagram p9: hidden frame]
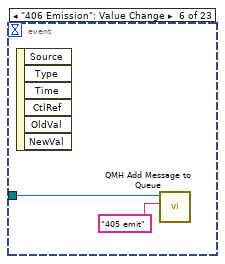
[diagram p10: hidden frame]
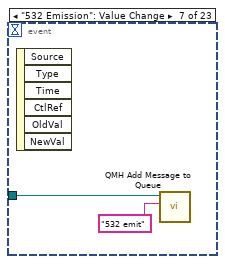
[diagram p11: hidden frame]
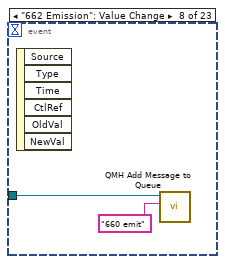
[diagram p12: hidden frame]
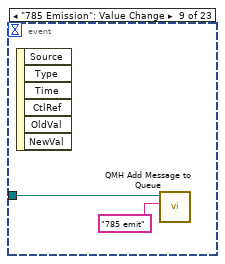
[diagram p13: hidden frame]
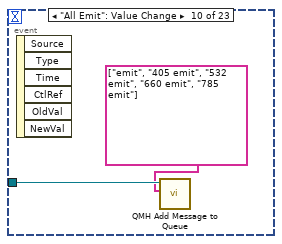
[diagram p14: hidden frame]
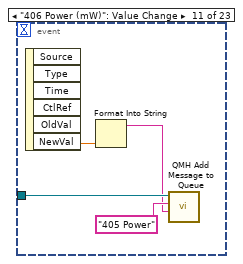
[diagram p15: hidden frame]
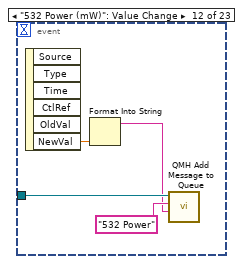
[diagram p16: hidden frame]
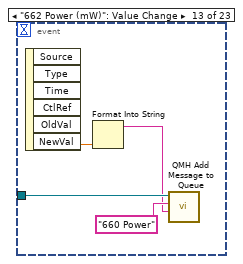
[diagram p17: hidden frame]
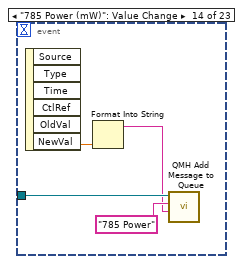
[diagram p18: hidden frame]
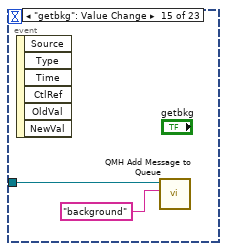
[diagram p19: hidden frame]
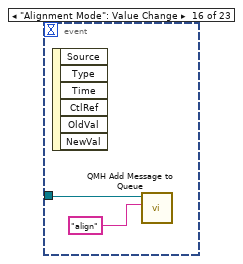
[diagram p20: hidden frame]
diagram:
  w47 = T8 {"# buffers"=10, "Buffer size"=44100, "unit (ms)"=enum."Samples"} ("Buffer")
  w46 = cluster{"Rate":i32, "Bits":i32, "Channels":i32} {"Rate"=44100, "Bits"=24, "Channels"=2} ("Format")
  w48 = u16 0 items=["Record", "Play", "Loopback", "ASIO input", "ASIO output"] ("Direction (Record)")
  w27 = dbl[] [1.0] ("X")
  # "PicoScope Acquire Rapid Block\nUses the PicoScope \"Acquire Rapid Block\" Method outlined in the PicoScope 2000 Series Programmers Guide, with decimation."
  # "Data acquisition is performed using the produce-consumer architecture for CRD."
  # "CRD Loops Below"
  # "Laser PAS Control Software\nSeptember 2016 (AF)"
  # "Laser PAS Control Software\nDecember 2016 (AF)"
  # "Data acquisition is performed using the produce-consumer architecture for both the microphone and photodiode.  One loop reads the data from the sound card and a parallel loop process the data."
  # "WaveIO from https://www.zeitnitz.eu/scms/waveio.\n(c) C. Zeitnitz 2015\nNo license is required for any private or public educational usage. If you plan a commercial application with WaveIO, please obtain a license."
  # "This loops adds messages to the queue to be processed in the message processor. In a UI application this loop typically uses the UI event structure to detect UI events and place them on the message queue. Other types of applcations may replace this structure with other code that will receive messages and place them on the queue.  The message processor reads messages and acts on them."
  # "Reset the Exit button"
  # "Unique Message\nQueue Name"
  # "Load initial messages\non the queue"
  # "DAQ/Processing Loops Below"
  # "UI Loops Below"
  n1 = Current VI's Path() -> (path=w92:path)
  n2 = Strip Path(path=w92) -> (name=w93:string)  [unwired: 1 out]
  n3 = call "QMH Create Queue.vi"("Initial Messages"=string[] ["Initialize"], "Message queue name (unnamed)"=w93) -> ("error out"=w89:errorcluster, "queue out"=w75:refnum<queue>)  [unwired: 8 in]
  n4 = while "Message Generator - User Interface Event Handler" {
    tunnel: w75 -> [w94]
    stop <- w95 stop-if-true
    w96 = 250  # Event Structure Timeout (ms)
    n5 = event shown="[17] \"set freqs\": Value Change" {
      selector: _ -> [_ _ _ _ _ _ _ _ _ _ _ _ _ _ _ _ _ _ _ _ _ _ _]
      dyn-events: _ -> [_ _ _ _ _ _ _ _ _ _ _ _ _ _ _ _ _ _ _ _ _ _ _]
      timeout: w96 -> [_ _ _ _ _ _ _ _ _ _ _ _ _ _ _ _ _ _ _ _ _ _ _]
      tunnel: [_ w99 TRUE ("Discard?") _ _ _ _ _ _ _ _ _ _ _ _ _ _ _ _ _ _ _ _] -> w95
      tunnel: w94 -> [_ w98 w101 w104 w108 w110 w112 w114 w116 w119 w122 w126 w130 w134 w136 w138 w141 w145 w150 w155 w159 w164 w166]
      event Timeout {
        n6 = event-data() -> ()  [unwired: 1 in, 1 out]
      }
      event Panel Close? {
        w99 = TRUE ("Discard?")
        # "Intercepts the upper right close panel\noperation to allow a smooth shutdown\nas opposed to immediately killing the app."
        n7 = event-data() -> ()  [unwired: 1 in, 3 out]
        n8 = call-poly "QMH Add Message to Queue.vi"("Message"="Exit", "queue in"=w98) -> ()  [unwired: 8 in, 2 out]
        n9 = event-data("Discard?"=w99) -> ()  [unwired: 1 in, 1 out]
      }
      event "Exit": Value Change {
        # "Exit the application\n>> Stop this message generator loop"
        n10 = event-data() -> ()  [unwired: 1 in, 6 out]
        n11 = call-poly "QMH Add Message to Queue.vi"("Message"="Exit", "queue in"=w101) -> ()  [unwired: 8 in, 2 out]
      }
      event Menu Selection (User) {
        # "Add run-time menu items to the message\nqueue. The message handler case names must match the menu ItemTag names."
        n12 = event-data() -> ("ItemTag"=w103:string)  [unwired: 1 in, 6 out]
        n13 = call-poly "QMH Add Message to Queue.vi"("Message"=w103, "queue in"=w104) -> ()  [unwired: 8 in, 2 out]
      }
      event "423 F (Hz)", "532 F (Hz)", "662 F (Hz)", "785 F (Hz)": Value Change {
        n14 = event-data() -> ("CtlRef"=w107:refnum<vi>)  [unwired: 1 in, 7 out]
        n15 = property class="DigNum (strict)"(reference=w107) -> (error out=w105:errorcluster, "Label.Text"=w106:string)  [unwired: 1 in, 1 out]
        n16 = call-poly "QMH Add Message to Queue.vi"("error in (no error)"=w105, "Parameter"=w106, "Message"="freqset", "queue in"=w108) -> ()  [unwired: 6 in, 2 out]
      }
      event "406 Emission": Value Change {
        n17 = event-data() -> ()  [unwired: 1 in, 6 out]
        n18 = call-poly "QMH Add Message to Queue.vi"("Message"="405 emit", "queue in"=w110) -> ()  [unwired: 8 in, 2 out]
      }
      event "532 Emission": Value Change {
        n19 = event-data() -> ()  [unwired: 1 in, 6 out]
        n20 = call-poly "QMH Add Message to Queue.vi"("Message"="532 emit", "queue in"=w112) -> ()  [unwired: 8 in, 2 out]
      }
      event "662 Emission": Value Change {
        n21 = event-data() -> ()  [unwired: 1 in, 6 out]
        n22 = call-poly "QMH Add Message to Queue.vi"("Message"="660 emit", "queue in"=w114) -> ()  [unwired: 8 in, 2 out]
      }
      event "785 Emission": Value Change {
        n23 = event-data() -> ()  [unwired: 1 in, 6 out]
        n24 = call-poly "QMH Add Message to Queue.vi"("Message"="785 emit", "queue in"=w116) -> ()  [unwired: 8 in, 2 out]
      }
      event "All Emit": Value Change {
        n25 = event-data() -> ()  [unwired: 1 in, 6 out]
        n26 = call-poly "QMH Add Message to Queue.vi"("Messages"=string[] ["emit", "405 emit", "532 emit", "660 emit", "785 emit"], "queue in"=w119) -> ()  [unwired: 8 in, 2 out]
      }
      event "406 Power (mW)": Value Change {
        n27 = event-data() -> ("NewVal"=w121:dbl)  [unwired: 1 in, 5 out]
        n28 = Format Into String(w121) -> (resulting string=w120:string)  [unwired: 3 in, 1 out]
        n29 = call-poly "QMH Add Message to Queue.vi"("Parameter"=w120, "Message"="405 Power", "queue in"=w122) -> ()  [unwired: 7 in, 2 out]
      }
      event "532 Power (mW)": Value Change {
        n30 = event-data() -> ("NewVal"=w125:dbl)  [unwired: 1 in, 5 out]
        n31 = Format Into String(w125) -> (resulting string=w124:string)  [unwired: 3 in, 1 out]
        n32 = call-poly "QMH Add Message to Queue.vi"("Parameter"=w124, "Message"="532 Power", "queue in"=w126) -> ()  [unwired: 7 in, 2 out]
      }
      event "662 Power (mW)": Value Change {
        n33 = event-data() -> ("NewVal"=w129:dbl)  [unwired: 1 in, 5 out]
        n34 = Format Into String(w129) -> (resulting string=w128:string)  [unwired: 3 in, 1 out]
        n35 = call-poly "QMH Add Message to Queue.vi"("Parameter"=w128, "Message"="660 Power", "queue in"=w130) -> ()  [unwired: 7 in, 2 out]
      }
      event "785 Power (mW)": Value Change {
        n36 = event-data() -> ("NewVal"=w133:dbl)  [unwired: 1 in, 5 out]
        n37 = Format Into String(w133) -> (resulting string=w132:string)  [unwired: 3 in, 1 out]
        n38 = call-poly "QMH Add Message to Queue.vi"("Parameter"=w132, "Message"="785 Power", "queue in"=w134) -> ()  [unwired: 7 in, 2 out]
      }
      event "getbkg": Value Change {
        n39 = event-data() -> ()  [unwired: 1 in, 6 out]
        n40 = call-poly "QMH Add Message to Queue.vi"("Message"="background", "queue in"=w136) -> ()  [unwired: 8 in, 2 out]
      }
      event "Alignment Mode": Value Change {
        n41 = event-data() -> ()  [unwired: 1 in, 6 out]
        n42 = call-poly "QMH Add Message to Queue.vi"("Message"="align", "queue in"=w138) -> ()  [unwired: 8 in, 2 out]
      }
      event "sweep": Value Change {
        n43 = event-data() -> ()  [unwired: 1 in, 6 out]
        n44 = call-poly "QMH Add Message to Queue.vi"("Message"="sweep", "queue in"=w141) -> ()  [unwired: 8 in, 2 out]
      }
      event "set freqs": Value Change {
        n45 = event-data() -> ()  [unwired: 1 in, 6 out]
        n46 = local read "Calculated Resonance (Hz)"() -> (w144:dbl)
        n47 = Format Into String(w144) -> (resulting string=w143:string, error out=w142:errorcluster)  [unwired: 3 in]
        n48 = call-poly "QMH Add Message to Queue.vi"("error in (no error)"=w142, "Parameter"=w143, "Message"="setfreqs", "queue in"=w145) -> ()  [unwired: 6 in, 2 out]
      }
      event "Save Data": Value Change {
        n49 = event-data() -> ("NewVal"=w149:bool)  [unwired: 1 in, 5 out]
        n50 = Format Into String(w149) -> (resulting string=w148:string, error out=w147:errorcluster)  [unwired: 3 in]
        n51 = call-poly "QMH Add Message to Queue.vi"("error in (no error)"=w147, "Parameter"=w148, "Message"="namefiles", "queue in"=w150) -> ()  [unwired: 6 in, 2 out]
      }
      event "Switch Filter": Value Change {
        n52 = event-data() -> ("NewVal"=w154:bool)  [unwired: 1 in, 5 out]
        n53 = local write "Filtering"(w154) -> ()
        n54 = Format Into String(w154) -> (resulting string=w152:string)  [unwired: 3 in, 1 out]
        n55 = call-poly "QMH Add Message to Queue.vi"("Parameter"=w152, "Message"="filterswitch", "queue in"=w155) -> ()  [unwired: 7 in, 2 out]
      }
      event "Time has Elapsed": Value Change {
        n56 = event-data() -> ("NewVal"=w158:bool)  [unwired: 1 in, 5 out]
        n57 = local read "Filtering"() -> (w157:bool)
        n58 = call "filterCreateMsg.vi"("time elapsed?"=w158, "auto sweep (true)"="Autosweep?", "filtering (true)"=w157, "queue in"=w159) -> ()  [unwired: 6 in, 2 out]
      }
      event "Calculated Resonance (Hz)": Value Change {
        n59 = event-data() -> ("NewVal"=w162:dbl)  [unwired: 1 in, 5 out]
        n60 = Format Into String(w162) -> (resulting string=w160:string, error out=w161:errorcluster)  [unwired: 3 in]
        n61 = call-poly "QMH Add Message to Queue.vi"("error in (no error)"=w161, "Parameter"=w160, "Message"="setfreqs", "queue in"=w164) -> ()  [unwired: 6 in, 2 out]
      }
      event "PAS Save": Value Change {
        n62 = event-data() -> ()  [unwired: 1 in, 6 out]
        n63 = call-poly "QMH Add Message to Queue.vi"("Message"="setwd", "queue in"=w166) -> ()  [unwired: 8 in, 2 out]
      }
    }
  }
  n64 = call <userlib>:"WaveIO_Open.vi"("Watchdog timeout (msec) (default=OFF)"=2000, "Format (44kHz, 16Bit, stereo)"=w46, "Buffer Config"=w47, "Direction (Record)"=w48, "idev"="mic id") -> ("error out"=w71:errorcluster, "Sound Handle Out"=w72:T9)  [unwired: 1 in]
  n65 = call <userlib>:"WaveIO_Open.vi"("Watchdog timeout (msec) (default=OFF)"=2000, "Format (44kHz, 16Bit, stereo)"=w46, "Buffer Config"=w47, "Direction (Record)"=w48, "idev"="pd id") -> ("error out"=w57:errorcluster, "Sound Handle Out"=w56:T9)  [unwired: 1 in]
  n66 = Obtain Queue(element data type="Data 2") -> (queue out=w40:refnum<queue>, error out=w78:errorcluster)  [unwired: 4 in, 1 out]
  n67 = Obtain Queue(element data type="Data 2") -> (queue out=w44:refnum<queue>, error out=w53:errorcluster)  [unwired: 4 in, 1 out]
  n68 = call <userlib>:"WaveIO_Start.vi"("error in (no error)"=w71, "Handle"=w72) -> ("error out"=w69:errorcluster, "Handle Out"=w70:T9)
  n69 = call <userlib>:"WaveIO_Start.vi"("error in (no error)"=w57, "Handle"=w56) -> ("error out"=w59:errorcluster, "Handle Out"=w58:T9)
  n70 = while {
    shift-right: [w175] -> w79
    shift-left: w40 -> [w173]
    shift-right: [w176] -> w80
    shift-left: w78 -> [w174]
    tunnel: w70 -> [w171]
    tunnel: w69 -> [w170]
    tunnel: [w168] -> w66
    tunnel: [w167] -> w65
    stop <- w172 stop-if-true
    # "Microphone DAQ Loop (Producer)"
    n71 = call <userlib>:"WaveIO_Record.vi"("Handle"=w171, "error in (no error)"=w170) -> ("Handle Out"=w168:T9, "Data"=w169:i32[][], "error out"=w167:errorcluster)  [unwired: 1 in, 2 out]
    n72 = local read "Exit"() -> (w172:bool)
    n73 = Enqueue Element(queue=w173, element=w169, error in (no error)=w174) -> (queue out=w175:refnum<queue>, error out=w176:errorcluster)  [unwired: 1 in, 1 out]
  }
  n74 = while {
    shift-right: [w185] -> w52
    shift-left: w44 -> [w183]
    shift-right: [w186] -> w51
    shift-left: w53 -> [w184]
    tunnel: w58 -> [w181]
    tunnel: w59 -> [w180]
    tunnel: [w178] -> w62
    tunnel: [w177] -> w63
    stop <- w182 stop-if-true
    # "PD DAQ Loop (Producer)"
    n75 = call <userlib>:"WaveIO_Record.vi"("Handle"=w181, "error in (no error)"=w180) -> ("Handle Out"=w178:T9, "Data"=w179:i32[][], "error out"=w177:errorcluster)  [unwired: 1 in, 2 out]
    n76 = local read "Exit"() -> (w182:bool)
    n77 = Enqueue Element(queue=w183, element=w179, error in (no error)=w184) -> (queue out=w185:refnum<queue>, error out=w186:errorcluster)  [unwired: 1 in, 1 out]
  }
  n78 = call <userlib>:"WaveIO_Stop.vi"("error in (no error)"=w65, "Handle"=w66) -> ("error out"=w67:errorcluster, "Handle Out"=w68:T9)
  n79 = Release Queue(queue=w79, error in (no error)=w80) -> (error out=w77:errorcluster)  [unwired: 1 in, 2 out]
  n80 = call <userlib>:"WaveIO_Stop.vi"("error in (no error)"=w63, "Handle"=w62) -> ("error out"=w61:errorcluster, "Handle Out"=w60:T9)
  n81 = Release Queue(queue=w52, error in (no error)=w51) -> (error out=w50:errorcluster)  [unwired: 1 in, 2 out]
  n82 = call <userlib>:"WaveIO_Close.vi"("error in (no error)"=w67, "Handle"=w68) -> ("error out"=w64:errorcluster)  [unwired: 1 out]
  n83 = call <userlib>:"WaveIO_Close.vi"("error in (no error)"=w61, "Handle"=w60) -> ("error out"=w49:errorcluster)  [unwired: 1 out]
  n84 = Divide(x=1.0, y=44100.0) -> (x/y=w41:dbl)
  n85 = Merge Errors(w64, w77, w49, w50) -> (w76:errorcluster)
  n86 = call "picoOpen.vi"() -> ("error out"=w24:errorcluster, "maxADC"=w6:i16, "Handle Out"=w25:i16)  [unwired: 8 in, 1 out]
  n87 = Obtain Queue(element data type=cluster{dbl, dbl, dbl, dbl} {0.0, 0.0, 0.0, 0.0}) -> (queue out=w30:refnum<queue>, error out=w34:errorcluster)  [unwired: 4 in, 1 out]
  n88 = Obtain Queue(element data type=cluster{dbl, dbl, dbl, dbl} {0.0, 0.0, 0.0, 0.0}) -> (queue out=w31:refnum<queue>, error out=w37:errorcluster)  [unwired: 4 in, 1 out]
  n89 = call "picoSetChannel.vi"("error in (no error)"=w24, "Channel B Settings"="Channel B Settings", "Channel A Settings"="Channel A Settings", "Handle Out"=w25) -> ("error out"=w11:errorcluster, "Handle Out"=w8:i16)  [unwired: 6 in]
  n90 = while {
    tunnel: w40 -> [w205]
    shift-right: [w202] -> _
    shift-left: w27 -> [w199]
    shift-right: [w201] -> _
    shift-left: w27 -> [w198]
    shift-right: [w200] -> _
    shift-left: w27 -> [w197]
    tunnel: w41 -> [w195]
    tunnel: "mic cal, scu" -> [w194]
    shift-right: [w192] -> w36
    shift-left: w31 -> [w191]
    shift-right: [w189] -> w35
    shift-left: w37 -> [w193]
    shift-right: [w187] -> _
    shift-left: w27 -> [w188]
    stop <- w196 stop-if-true
    # "Microphone Processing Loop (Consumer)"
    n91 = Dequeue Element(queue=w205) -> (element=w203:i32[][], error out=w204:errorcluster)  [unwired: 2 in, 2 out]
    n92 = case shown="No Error" w204 {
      selector: w204 -> [_ w247]
      tunnel: w203 -> [w239 _]
      tunnel: w199 -> [w243 w250]
      tunnel: w198 -> [w242 w248]
      tunnel: w197 -> [w241 w249]
      tunnel: [w216 w250] -> w202
      tunnel: [w215 w248] -> w201
      tunnel: [w214 w249] -> w200
      tunnel: [w223 w247] -> w196
      tunnel: w195 -> [w237 _]
      tunnel: w194 -> [w232 _]
      tunnel: [w217 T10 {"405 Mean"=0.0, "532 Mean"=0.0, "660 Mean"=0.0, "660 Mean 2"=0.0}] -> w190
      tunnel: w188 -> [w209 w245]
      tunnel: [w206 w245] -> w187
      frame No Error {
        w244 = T11 0 items=["Rectangle"=0, "Hanning"=1, "Hamming"=2, "Blackman-Harris"=3, "Exact Blackman"=4, "Blackman"=5, "Flat Top"=6, "4 Term B-Harris "=7, "7 Term B-Harris"=8, "Low Sidelobe"=9, "Blackman Nuttall"=11, "Triangle"=30, "Bartlett-Hanning"=31, "Bohman"=32, "Parzen"=33, "Welch"=34, "Kaiser"=60, "Dolph-Chebyshev"=61, "Gaussian"=62] ("window")
        n93 = Index Array(array=w239, index (row)=0) -> (element=w238:i32[])  [unwired: 1 in]
        n94 = Bundle By Name("Y"=w238, "dt"=w237) -> (w236:waveform(i32))  [unwired: 1 in]
        "micwave" <- w236
        n95 = local read "423 F (Hz)"() -> (w234:i32)
        n96 = local read "532 F (Hz)"() -> (w233:i32)
        n97 = local read "662 F (Hz)"() -> (w207:i32)
        n98 = local read "785 F (Hz)"() -> (w212:i32)
        n99 = call-poly <vilib>:"FFT Spectrum (Mag-Phase).vi"("window"=w244, "time signal"=w236) -> ("error out"=w224:errorcluster, "magnitude"=w235:cluster{"f0":dbl, "df":dbl, "magnitude":dbl[]})  [unwired: 5 in, 3 out]
        "micfft" <- w235
        n100 = call-poly "fftGetMagsPoly.vi"("input cluster"=w235, "405 F (Hz)"=w234, "532 F (Hz)"=w233, "660 F (Hz)"=w207, "785 F (Hz)"=w212, "unit cal, scu"=w232) -> ("mag405 (mV)"=w227:dbl, "mag532 (mV)"=w226:dbl, "mag660 (mV)"=w225:dbl, "mag785 (mV)"=w208:dbl)  [unwired: 6 in]
        n101 = Bundle("X"=w243, "mag405 (mV)"=w227) -> (w231:cluster{"X":dbl[], "mag405 (mV) ":dbl})  [unwired: 1 in]
        n102 = Bundle("X"=w242, "mag532 (mV)"=w226) -> (w230:cluster{"X":dbl[], "mag532 (mV)":dbl})  [unwired: 1 in]
        n103 = Bundle("X"=w241, "mag660 (mV)"=w225) -> (w229:cluster{"X":dbl[], "mag660 (mV)":dbl})  [unwired: 1 in]
        n104 = Bundle("X"=w209, "mag785 (mV)"=w208) -> (w210:cluster{"X":dbl[], "mag785 (mV)":dbl})  [unwired: 1 in]
        n105 = local read "PAS Save"() -> (w213:bool)
        n106 = local read "mic"() -> (w222:path)
        n107 = call-poly "rollingAverage_multi.vi"("Magnitude Averaging (no. Avgs.)"="rollavg", "785"=w210, "660"=w229, "532"=w230, "405"=w231) -> ("785 Data"=w211:T12, "660 Data"=w218:T13, "532 Data"=w219:T14, "405 Data"=w220:T15)  [unwired: 3 in]
        n108 = call "saveTimeSeries_IV.vi"("1"=w227, "file path (dialog if empty)"=w222, "save?"=w213, "2"=w226, "3"=w225, "4"=w208, "Error In"=w224, "Number of Data Series"=enum16{"1", "2", "3", "4"}."4") -> ("Error Out"=w223:errorcluster)  [unwired: 7 in]
        n109 = call-poly "micUnbundle.vi"("405nm Data"=w220, "532nm Data"=w219, "660nm Data"=w218, "785nm Data"=w211) -> ("pd ts"=w217:T7, "405 New Array"=w216:dbl[], "532 New Array"=w215:dbl[], "660 New Array"=w214:dbl[], "785 New Array"=w206:dbl[])  [unwired: 7 in]
        "mic ts" <- w217
      }
      frame Error {
      }
    }
    n110 = Enqueue Element(queue=w191, element=w190, error in (no error)=w193) -> (queue out=w192:refnum<queue>, error out=w189:errorcluster)  [unwired: 1 in, 1 out]
  }
  n111 = while {
    shift-right: [w271] -> _
    shift-left: w27 -> [w268]
    shift-right: [w270] -> _
    shift-left: w27 -> [w267]
    shift-right: [w269] -> _
    shift-left: w27 -> [w266]
    tunnel: w44 -> [w264]
    tunnel: w41 -> [w263]
    tunnel: "mic cal, scu" -> [w262]
    shift-right: [w259] -> w33
    shift-left: w30 -> [w260]
    shift-right: [w258] -> w32
    shift-left: w34 -> [w261]
    shift-right: [w251] -> _
    shift-left: w27 -> [w253]
    stop <- w265 stop-if-true
    # "Photodiode Processing Loop (Consumer)"
    n112 = Dequeue Element(queue=w264) -> (element=w272:i32[][], error out=w273:errorcluster)  [unwired: 2 in, 2 out]
    n113 = case shown="No Error" w273 {
      selector: w273 -> [_ w319]
      tunnel: w272 -> [w311 _]
      tunnel: w268 -> [w315 w322]
      tunnel: w267 -> [w314 w320]
      tunnel: w266 -> [w313 w321]
      tunnel: [w287 w322] -> w271
      tunnel: [w286 w320] -> w270
      tunnel: [w285 w321] -> w269
      tunnel: [w295 w319] -> w265
      tunnel: w263 -> [w309 _]
      tunnel: w262 -> [w304 _]
      tunnel: "660 PD Cal 3" -> [w282 _]
      tunnel: "532 PD Cal 3" -> [w283 _]
      tunnel: "405 PD Cal 3" -> [w284 _]
      tunnel: [w288 cluster{dbl, dbl, dbl, dbl} {0.0, 0.0, 0.0, 0.0}] -> w257
      tunnel: w253 -> [w280 w317]
      tunnel: "785 PD Cal" -> [w277 _]
      tunnel: [w275 w317] -> w251
      frame No Error {
        w316 = T11 0 items=["Rectangle"=0, "Hanning"=1, "Hamming"=2, "Blackman-Harris"=3, "Exact Blackman"=4, "Blackman"=5, "Flat Top"=6, "4 Term B-Harris "=7, "7 Term B-Harris"=8, "Low Sidelobe"=9, "Blackman Nuttall"=11, "Triangle"=30, "Bartlett-Hanning"=31, "Bohman"=32, "Parzen"=33, "Welch"=34, "Kaiser"=60, "Dolph-Chebyshev"=61, "Gaussian"=62] ("window")
        n114 = Index Array(array=w311, index (row)=0) -> (element=w310:i32[])  [unwired: 1 in]
        n115 = Bundle By Name("Y"=w310, "dt"=w309) -> (w308:waveform(i32))  [unwired: 1 in]
        "pdwave" <- w308
        n116 = local read "423 F (Hz)"() -> (w306:i32)
        n117 = local read "532 F (Hz)"() -> (w305:i32)
        n118 = local read "662 F (Hz)"() -> (w276:i32)
        n119 = local read "785 F (Hz)"() -> (w279:i32)
        n120 = call-poly <vilib>:"FFT Spectrum (Mag-Phase).vi"("window"=w316, "time signal"=w308) -> ("error out"=w296:errorcluster, "magnitude"=w307:cluster{"f0":dbl, "df":dbl, "magnitude":dbl[]})  [unwired: 5 in, 3 out]
        "pdfft" <- w307
        n121 = call-poly "fftGetMagsPoly.vi"("input cluster"=w307, "405 F (Hz)"=w306, "532 F (Hz)"=w305, "660 F (Hz)"=w276, "785 F (Hz)"=w279, "unit cal, scu"=w304) -> ("mag405 (mV)"=w299:dbl, "mag532 (mV)"=w298:dbl, "mag660 (mV)"=w297:dbl, "mag785 (mV)"=w274:dbl)  [unwired: 6 in]
        n122 = Bundle("X"=w315, "mag405 (mV)"=w299) -> (w303:cluster{"X":dbl[], "mag405 (mV) ":dbl})  [unwired: 1 in]
        n123 = Bundle("X"=w314, "mag532 (mV)"=w298) -> (w302:cluster{"X":dbl[], "mag532 (mV)":dbl})  [unwired: 1 in]
        n124 = Bundle("X"=w313, "mag660 (mV)"=w297) -> (w301:cluster{"X":dbl[], "mag660 (mV)":dbl})  [unwired: 1 in]
        n125 = Bundle("X"=w280, "mag785 (mV)"=w274) -> (w281:cluster{"X":dbl[], "mag785 (mV)":dbl})  [unwired: 1 in]
        n126 = local read "PAS Save"() -> (w294:bool)
        n127 = local read "pd"() -> (w293:path)
        n128 = call-poly "rollingAverage_multi.vi"("Magnitude Averaging (no. Avgs.)"="Chart Rolling Average", "785"=w281, "660"=w301, "532"=w302, "405"=w303) -> ("785 Data"=w278:T12, "660 Data"=w289:T13, "532 Data"=w290:T14, "405 Data"=w291:T15)  [unwired: 3 in]
        n129 = call "saveTimeSeries_IV.vi"("1"=w299, "file path (dialog if empty)"=w293, "save?"=w294, "2"=w298, "3"=w297, "4"=w274, "Error In"=w296, "Number of Data Series"=enum16{"1", "2", "3", "4"}."4") -> ("Error Out"=w295:errorcluster)  [unwired: 7 in]
        n130 = call-poly "pdNormalize.vi"("405 Data"=w291, "532 Data"=w290, "660 Data"=w289, "785 Data"=w278, "785 PD Cal"=w277, "405 PD Cal"=w284, "532 PD Cal"=w283, "660 PD Cal"=w282) -> ("Output Cluster"=w288:cluster{dbl, dbl, dbl, dbl}, "405 New Array"=w287:dbl[], "532 New Array"=w286:dbl[], "660 New Array"=w285:dbl[], "785 New Array"=w275:dbl[])  [unwired: 3 in]
        "pd ts" <- w288
      }
      frame Error {
      }
    }
    n131 = Enqueue Element(queue=w260, element=w257, error in (no error)=w261) -> (queue out=w259:refnum<queue>, error out=w258:errorcluster)  [unwired: 1 in, 1 out]
  }
  n132 = while {
    tunnel: w31 -> [w324]
    tunnel: w30 -> [w323]
    stop <- w329 stop-if-true
    # "This loop takes data from the two FFT loops and converts to absorption via the calibration."
    # "Absorption Data Loop (Consummer II)"
    n133 = Dequeue Element(queue=w324) -> (element=w330:cluster{dbl, dbl, dbl, dbl}, error out=w328:errorcluster)  [unwired: 2 in, 2 out]
    n134 = Dequeue Element(queue=w323) -> (element=w325:cluster{dbl, dbl, dbl, dbl}, error out=w327:errorcluster)  [unwired: 2 in, 2 out]
    n135 = Merge Errors(w328, w327) -> (w326:errorcluster)
    n136 = case shown="No Error" w326 {
      selector: w326 -> [w341 w343]
      tunnel: w330 -> [w333 _]
      tunnel: [w340 w343] -> w329
      tunnel: w325 -> [w332 _]
      frame No Error {
        n137 = local read "processed"() -> (w337:path)
        n138 = local read "PAS Save"() -> (w338:bool)
        n139 = local read "tau"() -> (w331:dbl)
        n140 = call-poly "absCalcPlot.vi"("crd"=w331, "file path (dialog if empty)"=w337, "Cell Calibration, mV/mW"="cellcal", "save?"=w338, "Error In"=w341, "PD Values"=w332, "bkg values"="Bkg Values (mV)", "Mic Values"=w333) -> ("Error Out"=w340:errorcluster, "aae"=→"AAE":dbl, "b_abs/ext ts"=→"abs/ext":cluster{dbl, dbl, dbl, dbl, "crd":dbl}, "Spectrum"=→"Absorption Spectrum":cluster{dbl[], "Best Power Fit":dbl[]}[])
      }
      frame Error {
      }
    }
  }
  n141 = while "Message Processor" {
    shift-left: w89 -> [w357]
    shift-right: [w349] -> w85
    tunnel: w75 -> [w356]
    shift-left: "State Variables" -> [w362]
    shift-right: [w361] -> _
    tunnel: "406 Port" -> [w353]
    tunnel: "532 Port" -> [w352]
    tunnel: "662 Port" -> [w351]
    tunnel: "Teensy Port" -> [w350]
    shift-right: [w347] -> _
    shift-left: _ -> [w346]
    tunnel: "785 Port" -> [w344]
    stop <- w360 stop-if-true
    w354 = 100  # Timeout
    n142 = call "QMH Get Next Message from Queue.vi"("error in (no error)"=w357, "ms timeout (1)"=w354, "queue in"=w356) -> ("error out"=w358:errorcluster, "Next Parameter"=w345:string, "Next Message"=w355:string, "queue out"=w359:refnum<queue>, "Stop QMH"=w360:bool)  [unwired: 3 in]
    n143 = case shown="\"filter\"" w355 {
      selector: w355 -> [_ w390 _ _ _ _ _ _ _ _ _ _ _ _ _ _ _ _ _ _ _ _]
      tunnel: [w386 w391 w406 w417 w480 w511 w513 w520 w526 w532 w538 w544 w552 w559 w566 w573 w594 w601 w626 w637 w650 w662] -> w361
      tunnel: w362 -> [w386 w391 w406 w417 w480 w511 w513 w520 w526 w532 w538 w544 w552 w559 w566 w573 w594 w601 w626 w637 w650 w662]
      tunnel: w359 -> [_ _ _ w410 _ _ _ _ _ _ _ _ _ _ _ _ _ _ _ _ w648 w663]
      tunnel: w358 -> [w378 w387 w404 w416 w478 w510 w516 w522 w528 w534 w537 w540 w549 w556 w564 w571 w595 w598 w624 w636 w649 w664]
      tunnel: [w374 w387 w397 w409 w477 w506 w512 w518 w524 w531 w537 w543 w550 w557 w565 w567 w595 w597 w623 w636 w646 w653] -> w349
      tunnel: w353 -> [w380 _ w405 w408 _ _ w515 _ _ _ _ w545 _ _ _ w570 _ _ _ _ _ w659]
      tunnel: w352 -> [w379 _ w402 w412 _ _ _ w519 _ _ _ _ w551 _ _ w569 _ _ _ _ _ w658]
      tunnel: w351 -> [w373 _ w401 w415 _ _ _ _ w525 _ _ _ _ w558 _ w568 _ _ _ _ _ w657]
      tunnel: w350 -> [_ _ w399 w411 w479 w505 _ _ _ _ _ _ _ _ _ _ _ w599 w625 _ _ w660]
      tunnel: w345 -> [_ _ _ _ w476 w509 _ _ _ _ _ w542 w546 w553 w561 _ _ _ w622 w635 _ _]
      tunnel: w344 -> [w377 _ w392 w407 _ _ _ _ _ w530 _ _ _ _ w560 _ _ _ _ _ _ w651]
      frame "", "Wait" {
        # "Update the front panel"
        # "Idle Case - this case is called after a Timeout on the Get Next Message from Queue VI, if no new messages are present on the queue. This case can be used for housekeeping tasks such as updating the UI."
        n144 = Get Date/Time String(want seconds? (F)=TRUE) -> (date string=w385:string, time string=w384:string)  [unwired: 2 in]
        n145 = call-poly "laserDiagnose.vi"("405 Port"=w380, "532 Port"=w379, "660 Port"=w373, "785 Port"=w377, "error in (no error)"=w378) -> ("Temperatures"=→"Laser Temperatures":T3, "Overtemp"=→"Overtemp":bool, "error out"=w374:errorcluster)  [unwired: 6 in, 2 out]
        n146 = Concatenate Strings(w385, " " ("string"), w384) -> (→"Status":string)
      }
      frame Default {
        # "Call this case if a message is received that is not handled \nby any other case. Typically this is a programming error\nas a result of a typo or unhandled message/missing message handler."
        n147 = Format Into String(format string="DevError: Missing message handler for '%s\" message." ("message"), w390) -> (resulting string=w388:string)  [unwired: 2 in, 1 out]
        n148 = One Button Dialog(message=w388) -> ()  [unwired: 1 in, 1 out]
      }
      frame "Initialize" {
        w393 = u32 115200 ("baud rate (9600)")
        # "Initialize the state variables and user interface\nInitialize serial connections"
        n149 = call-poly "VISA Configure Serial Port"("VISA resource name"=w405, "baud rate (9600)"=w393, "error in (no error)"=w404) -> ("error out"=w403:errorcluster)  [unwired: 11 in, 1 out]
        n150 = call-poly "VISA Configure Serial Port"("VISA resource name"=w402, "baud rate (9600)"=w393, "error in (no error)"=w403) -> ("error out"=w400:errorcluster)  [unwired: 11 in, 1 out]
        n151 = call-poly "VISA Configure Serial Port"("VISA resource name"=w401, "baud rate (9600)"=w393, "error in (no error)"=w400) -> ("error out"=w395:errorcluster)  [unwired: 11 in, 1 out]
        n152 = call-poly "VISA Configure Serial Port"("VISA resource name"=w392, "baud rate (9600)"=w393, "error in (no error)"=w395) -> ("error out"=w394:errorcluster)  [unwired: 11 in, 1 out]
        n153 = call-poly "VISA Configure Serial Port"("VISA resource name"=w399, "error in (no error)"=w394) -> ("VISA resource name out"=w398:refnum<visa-resource-name>, "error out"=w396:errorcluster)  [unwired: 12 in]
        n154 = property class="Instr" props=["Baud"](reference=w398, error in=w396) -> (error out=w397:errorcluster)  [unwired: 2 out]
      }
      frame "sweep" {
        # "Perform a frequency sweep and calculate the resonance frequency"
        n155 = stacked-sequence {
          seq-local: [_ w432 _ _] -> [_ _ w460 _]
          tunnel: w416 -> [_ w426 _ _]
          tunnel: "Data End Frequency (Hz)" -> [_ w429 w454 _]
          tunnel: "Data Start Frequency (Hz)" -> [_ w428 w453 _]
          tunnel: w415 -> [w423 _ _ w470]
          tunnel: w412 -> [w421 _ _ w469]
          tunnel: w411 -> [_ w427 _ _]
          tunnel: w410 -> [_ _ _ w474]
          tunnel: [_ _ _ w471] -> w409
          tunnel: w408 -> [_ _ _ _]
          tunnel: w407 -> [w418 _ _ w465]
          frame #0 {
            w419 = FALSE
            # "Turn red, green, IR lasers off for scan."
            n156 = call "laserOnOff.vi"("Emission (F = OFF)"=w419, "VISA Refnum in"=w421) -> ("error out"=w425:errorcluster)  [unwired: 7 in, 2 out]
            n157 = Wait (ms)(milliseconds to wait=u32 5000) -> ()  [unwired: 1 out]
            n158 = local write "Status"("Conducting Frequency Sweep" ("Status")) -> ()
            n159 = call "laserOnOff.vi"("error in (no error)"=w425, "Emission (F = OFF)"=w419, "VISA Refnum in"=w423) -> ("error out"=w420:errorcluster)  [unwired: 6 in, 2 out]
            n160 = call "laserOnOff.vi"("error in (no error)"=w420, "Emission (F = OFF)"=w419, "VISA Refnum in"=w418) -> ()  [unwired: 6 in, 3 out]
          }
          frame #1 {
            n161 = Subtract(x=w429, y=w428) -> (x-y=w430:i32)
            n162 = for {
              N: w430 -> [w436]
              tunnel: [w441] -> w432 mode=indexing
              tunnel: w428 -> [w440]
              tunnel: w429 -> [w439]
              tunnel: w426 -> [_]
              i -> [w433]
              # "Get microphone data."
              # "Listen for N*2000\n seconds"
              n163 = Increment(x=w433) -> (x+1=w434:i32)
              n164 = Divide(x=w434, y=w436) -> (x/y=→"sweep progress":dbl)
              n165 = local read "micfft"() -> (w438:cluster{"f0":dbl, "df":dbl, "magnitude":dbl[]})
              n166 = Unbundle By Name(w438) -> ("magnitude"=w437:dbl[])
              n167 = Wait (ms)(milliseconds to wait=u32 2000) -> ()  [unwired: 1 out]
              n168 = call "fftGetMax.vi"("End Frequency (Hz)"=w439, "Start Frequency (Hz)"=w440, "Magnitudes"=w437) -> ("max value"=w441:dbl)  [unwired: 8 in]
            }
            n169 = case shown="False" TRUE ("sweep?") {
              tunnel: w428 -> [_ w448]
              tunnel: w429 -> [_ w447]
              tunnel: w427 -> [_ w446]
              tunnel: [w443 w445] -> _
              tunnel: w426 -> [w443 w444]
              frame False {
              }
              frame True {
                # "Scan laser freq.\nwith Teensy"
                n170 = call "teensySweepFreq.vi"("error in (no error)"=w444, "end f, Hz (1385)"=w447, "start f, Hz (1355)"=w448, "VISA Refnum in"=w446) -> ("error out"=w445:errorcluster)  [unwired: 7 in]
              }
            }
          }
          frame #2 {
            # "Calculate resonance frequency;\ndisplay and save scan."
            n171 = Wait (ms)(milliseconds to wait=u32 5000) -> ()  [unwired: 1 out]
            n172 = local read "PAS Save"() -> (w449:bool)
            n173 = To Double Precision Float(number=w454) -> (double precision float=w451:dbl)
            n174 = To Double Precision Float(number=w453) -> (double precision float=w452:dbl)
            n175 = call "resCalc.vi"("Frequency Sweep"=w460, "Start F, Hz (1355)"=w453) -> ("F-res, Hz"=w458:dbl, "Frequency Scan"=w450:cluster{i32[], "Best Gaussian Fit":dbl[]}[])  [unwired: 8 in]
            "freqscan" <- w450
            n176 = In Range and Coerce(upper limit=w451, x=w458, lower limit=w452) -> (In Range?=w457:bool)  [unwired: 1 out]
            n177 = case shown="True" w449 {
              tunnel: w450 -> [_ w464]
              tunnel: w458 -> [_ w463]
              frame False {
              }
              frame True {
                n178 = local read "sweeps"() -> (w462:path)
                n179 = call "saveFreqSweep.vi"("f-res, Hz"=w463, "Frequency Scan"=w464, "file path (dialog if empty)"=w462) -> ()  [unwired: 9 in]
              }
            }
            n180 = And(x=w457, y=TRUE ("check freqs?")) -> (x .and. y?=w455:bool)
            n181 = case shown="True" w455 {
              tunnel: w458 -> [_ w461]
              frame False {
              }
              frame True {
                n182 = property on="Calculated Resonance (Hz)" class="DigNum (strict)"("Val(Sgnl)"=w461) -> ()  [unwired: 2 in, 2 out]
                "Calculated Resonance (Hz)" <- w461
              }
            }
          }
          frame #3 {
            w466 = TRUE
            # "Turn red, green, IR lasers back on."
            n183 = call "laserOnOff.vi"("Emission (F = OFF)"=w466, "VISA Refnum in"=w469) -> ("error out"=w475:errorcluster)  [unwired: 7 in, 2 out]
            n184 = call "laserOnOff.vi"("error in (no error)"=w475, "Emission (F = OFF)"=w466, "VISA Refnum in"=w470) -> ("error out"=w468:errorcluster)  [unwired: 6 in, 2 out]
            n185 = call "laserOnOff.vi"("error in (no error)"=w468, "Emission (F = OFF)"=w466, "VISA Refnum in"=w465) -> ("error out"=w467:errorcluster)  [unwired: 6 in, 2 out]
            n186 = call-poly "QMH Add Message to Queue.vi"("error in (no error)"=w467, "Parameter"="532 F (Hz)", "Message"="freqset", "queue in"=w474) -> ("error out"=w471:errorcluster)  [unwired: 6 in, 1 out]
          }
        }
      }
      frame "freqset" {
        # "Set the frequency of the Teensy's modulation\nsignal for single laser (if single frequency is changed)."
        # "Set the laser frequency.  Case for \"red\", \"blue\", or \"green\"."
        n187 = case shown="\"405 F (Hz) \", Default" w476 {
          tunnel: w478 -> [w485 w490 w494 w500]
          tunnel: [w484 w489 w493 w499] -> w477
          tunnel: w479 -> [w481 w486 w491 w498]
          frame "405 F (Hz) ", Default {
            w483 = u16 0 items=["blue", "green", "red"] ("laser")
            n188 = call "freqSet.vi"("error in (no error)"=w485, "laser"=w483, "Freq, Hz (1370)"="423 F (Hz)", "Teensy Port"=w481) -> ("error out"=w484:errorcluster)  [unwired: 6 in, 1 out]
          }
          frame "532 F (Hz)" {
            w488 = u16 1 items=["blue", "green", "red"] ("laser")
            n189 = call "freqSet.vi"("error in (no error)"=w490, "laser"=w488, "Freq, Hz (1370)"="532 F (Hz)", "Teensy Port"=w486) -> ("error out"=w489:errorcluster)  [unwired: 6 in, 1 out]
          }
          frame "662 F (Hz)" {
            w495 = u16 2 items=["blue", "green", "red"] ("laser")
            n190 = call "freqSet.vi"("error in (no error)"=w494, "laser"=w495, "Freq, Hz (1370)"="662 F (Hz)", "Teensy Port"=w491) -> ("error out"=w493:errorcluster)  [unwired: 6 in, 1 out]
          }
          frame "785 F (Hz)" {
            w496 = u16 3 items=["blue", "green", "red", "ir"] ("laser")
            n191 = call "freqSet.vi"("error in (no error)"=w500, "laser"=w496, "Freq, Hz (1370)"="785 F (Hz)", "Teensy Port"=w498) -> ("error out"=w499:errorcluster)  [unwired: 6 in, 1 out]
          }
        }
      }
      frame "setfreqs" {
        # "Set the frequency of the Teensy's modulation\nsignal for all lasers at once."
        # "Set laser frequencies to resonance frequency calculated in sweep."
        n192 = Scan From String(input string=w509, error in=w510) -> (error out=w507:errorcluster, output 1=w508:dbl)  [unwired: 3 in, 2 out]
        n193 = call-poly "lasersSetFrequencies.vi"("VISA Refnum in"=w505, "f-res (Hz)"=w508, "error in (no error)"=w507) -> ("405 f (Hz)"=w504:i32, "532 f (Hz)"=w503:i32, "662 f (Hz)"=w502:i32, "785 f (Hz)"=w501:i32, "error out"=w506:errorcluster)  [unwired: 8 in]
        n194 = local write "662 F (Hz)"(w502) -> ()
        n195 = local write "532 F (Hz)"(w503) -> ()
        n196 = local write "423 F (Hz)"(w504) -> ()
        n197 = local write "785 F (Hz)"(w501) -> ()
      }
      frame "405 emit" {
        # "Turn laser on or off"
        n198 = call "laserOnOff.vi"("error in (no error)"=w516, "Emission (F = OFF)"="406 Emission", "Power, mW (100)"="406 Power (mW)", "VISA Refnum in"=w515) -> ("error out"=w512:errorcluster)  [unwired: 5 in, 2 out]
      }
      frame "532 emit" {
        # "Turn laser on or off"
        n199 = call "laserOnOff.vi"("error in (no error)"=w522, "Emission (F = OFF)"="532 Emission", "Power, mW (100)"="532 Power (mW)", "VISA Refnum in"=w519) -> ("error out"=w518:errorcluster)  [unwired: 5 in, 2 out]
      }
      frame "660 emit" {
        # "Turn laser on or off"
        n200 = call "laserOnOff.vi"("error in (no error)"=w528, "Emission (F = OFF)"="662 Emission", "Power, mW (100)"="662 Power (mW)", "VISA Refnum in"=w525) -> ("error out"=w524:errorcluster)  [unwired: 5 in, 2 out]
      }
      frame "785 emit" {
        # "Turn laser on or off"
        n201 = call "laserOnOff.vi"("error in (no error)"=w534, "Emission (F = OFF)"="785 Emission", "Power, mW (100)"="785 Power (mW)", "VISA Refnum in"=w530) -> ("error out"=w531:errorcluster)  [unwired: 5 in, 2 out]
      }
      frame "emit" {
        # "Turn on all lasers."
        n202 = local write "406 Emission"("All Emit") -> ()
        n203 = local write "532 Emission"("All Emit") -> ()
        n204 = local write "662 Emission"("All Emit") -> ()
        n205 = local write "785 Emission"("All Emit") -> ()
      }
      frame "405 Power" {
        # "Set laser power"
        n206 = Scan From String(input string=w542, error in=w540) -> (error out=w539:errorcluster, output 1=w541:dbl)  [unwired: 3 in, 2 out]
        n207 = call "laserSetPower.vi"("error in (no error)"=w539, "Laser Power (mW)"=w541, "VISA Refnum in"=w545) -> ("error out"=w543:errorcluster)  [unwired: 7 in, 1 out]
      }
      frame "532 Power" {
        n208 = Scan From String(input string=w546, error in=w549) -> (error out=w548:errorcluster, output 1=w547:dbl)  [unwired: 3 in, 2 out]
        n209 = call "laserSetPower.vi"("error in (no error)"=w548, "Laser Power (mW)"=w547, "VISA Refnum in"=w551) -> ("error out"=w550:errorcluster)  [unwired: 7 in, 1 out]
      }
      frame "660 Power" {
        n210 = Scan From String(input string=w553, error in=w556) -> (error out=w555:errorcluster, output 1=w554:dbl)  [unwired: 3 in, 2 out]
        n211 = call "laserSetPower.vi"("error in (no error)"=w555, "Laser Power (mW)"=w554, "VISA Refnum in"=w558) -> ("error out"=w557:errorcluster)  [unwired: 7 in, 1 out]
      }
      frame "785 Power" {
        n212 = Scan From String(input string=w561, error in=w564) -> (error out=w563:errorcluster, output 1=w562:dbl)  [unwired: 3 in, 2 out]
        n213 = call "laserSetPower.vi"("error in (no error)"=w563, "Laser Power (mW)"=w562, "VISA Refnum in"=w560) -> ("error out"=w565:errorcluster)  [unwired: 7 in, 1 out]
      }
      frame "align" {
        # "Set power of all lasers to 5 mW for alignment"
        n214 = case shown="True" "Alignment Mode" {
          tunnel: w571 -> [w581 w591]
          tunnel: w570 -> [w580 w590]
          tunnel: w569 -> [w579 w589]
          tunnel: w568 -> [w578 w588]
          tunnel: [w575 w585] -> w567
          frame True {
            w574 = 5.0 ("Laser Power (mW)")
            n215 = call "laserSetPower.vi"("error in (no error)"=w581, "Laser Power (mW)"=w574, "VISA Refnum in"=w580) -> ("error out"=w577:errorcluster)  [unwired: 7 in, 1 out]
            n216 = call "laserSetPower.vi"("error in (no error)"=w577, "Laser Power (mW)"=w574, "VISA Refnum in"=w579) -> ("error out"=w576:errorcluster)  [unwired: 7 in, 1 out]
            n217 = call "laserSetPower.vi"("error in (no error)"=w576, "Laser Power (mW)"=w574, "VISA Refnum in"=w578) -> ("error out"=w575:errorcluster)  [unwired: 7 in, 1 out]
          }
          frame False, Default {
            n218 = local read "406 Power (mW)"() -> (w584:dbl)
            n219 = local read "532 Power (mW)"() -> (w583:dbl)
            n220 = local read "662 Power (mW)"() -> (w582:dbl)
            n221 = call "laserSetPower.vi"("error in (no error)"=w591, "Laser Power (mW)"=w584, "VISA Refnum in"=w590) -> ("error out"=w587:errorcluster)  [unwired: 7 in, 1 out]
            n222 = call "laserSetPower.vi"("error in (no error)"=w587, "Laser Power (mW)"=w583, "VISA Refnum in"=w589) -> ("error out"=w586:errorcluster)  [unwired: 7 in, 1 out]
            n223 = call "laserSetPower.vi"("error in (no error)"=w586, "Laser Power (mW)"=w582, "VISA Refnum in"=w588) -> ("error out"=w585:errorcluster)  [unwired: 7 in, 1 out]
          }
        }
      }
      frame "background" {
        n224 = local read "mic ts"() -> (w593:T7)
        n225 = local read "tau"() -> (w592:dbl)
        n226 = local write "Bkg Values (mV)"(w593) -> ()
        n227 = local write "tau0"(w592) -> ()
      }
      frame "filter" {
        n228 = local read "Filtering"() -> (w600:bool)
        n229 = case shown="True" w600 {
          tunnel: w599 -> [w604 w613]
          tunnel: w598 -> [w603 w611]
          tunnel: [w602 w612] -> w597
          frame False {
            n230 = Multiply(x="Filter Length (min)", y=60.0) -> (x*y=w607:dbl)
            n231 = local write "Time Target (s)"(w607) -> ()
            n232 = VISA Write(VISA resource name=w604, write buffer="v.1", error in (no error)=w603) -> (error out=w602:errorcluster)  [unwired: 2 out]
            "Filtering" <- TRUE
          }
          frame True {
            n233 = flat-sequence {
              tunnel: w611 -> [w621]
              tunnel: [w621] -> w610
              frame #0 {
                n234 = local read "tau"() -> (w619:dbl)
                n235 = local read "mic ts"() -> (w620:T7)
                n236 = local write "Bkg Values (mV)"(w620) -> ()
                n237 = local write "tau0"(w619) -> ()
              }
            }
            n238 = local write "Filtering"(FALSE) -> ()
            n239 = VISA Write(VISA resource name=w613, write buffer="v.0", error in (no error)=w610) -> (error out=w612:errorcluster)  [unwired: 2 out]
            n240 = Multiply(x="Sample Length (min)", y=60.0) -> (x*y=w615:dbl)
            n241 = local write "Time Target (s)"(w615) -> ()
          }
        }
        n242 = Wait (ms)(milliseconds to wait=u32 500) -> ()  [unwired: 1 out]
      }
      frame "filterswitch" {
        n243 = case shown="\"TRUE\"" w622 {
          tunnel: w625 -> [w629 w634]
          tunnel: w624 -> [w628 w633]
          tunnel: [w627 w632] -> w623
          frame "FALSE", Default {
            n244 = VISA Write(VISA resource name=w629, write buffer="v.0", error in (no error)=w628) -> (error out=w627:errorcluster)  [unwired: 2 out]
          }
          frame "TRUE" {
            n245 = VISA Write(VISA resource name=w634, write buffer="v.1", error in (no error)=w633) -> (error out=w632:errorcluster)  [unwired: 2 out]
          }
        }
      }
      frame "namefiles" {
        n246 = case shown="\"TRUE\"" w635 {
          frame "FALSE", Default {
            n247 = local write "PAS Save"(FALSE ("PAS Save")) -> ()
          }
          frame "TRUE" {
            n248 = flat-sequence {
              frame #0 {
                n249 = call "saveSetDirectory.vi"() -> ("mic"=→"mic":path, "pd"=→"pd":path, "processed"=→"processed":path, "sweeps"=→"sweeps":path, "crd"=→"crd":path)  [unwired: 11 in]
              }
              frame #1 {
                "PAS Save" <- TRUE ("PAS Save")
              }
            }
          }
        }
      }
      frame "Error" {
        (unwired) errorcluster {"status"=FALSE, "code"=0, "source"=""} ("error out")
        # "Proceed to Exit - remove if this is\nnot appropriate for the General Error case"
        # "General Error Case - this case is called if an error is passed using the error cluster below. Typically most new errors should be handed in each individual case and not passed in the rror cluster. If necessary a custom error handler case should be added and called from other cases."
        n250 = call <vilib>:"Simple Error Handler.vi"("error in (no error)"=w649) -> ("error out"=w645:errorcluster)  [unwired: 4 in, 4 out]
        n251 = call-poly "QMH Add Message to Queue.vi"("error in (no error)"=w645, "Message"="Exit", "queue in"=w648) -> ("error out"=w646:errorcluster)  [unwired: 7 in, 1 out]
      }
      frame "Exit" {
        # "Perform cleanup tasks: Close serial connections and clear front panel."
        n252 = call "QMH Destroy Queue.vi"("error in (no error)"=w664, "queue in"=w663) -> ("error out"=w656:errorcluster)  [unwired: 7 in, 2 out]
        n253 = for {
          N: 4 -> [_]
          tunnel: w659 -> [w672]
          tunnel: w658 -> [w670]
          tunnel: w657 -> [w669]
          tunnel: w656 -> [w668]
          tunnel: FALSE -> [w667]
          tunnel: [w666] -> w652
          tunnel: w651 -> [w665]
          i -> [w671]
          # "Close laser serial connections."
          n254 = case shown="0, Default" w671 {
            tunnel: [w679 w684 w689 w694] -> w674
            tunnel: [w678 w683 w688 w693] -> w673
            tunnel: w672 -> [w677 _ _ _]
            tunnel: w670 -> [_ w682 _ _]
            tunnel: w669 -> [_ _ w686 _]
            tunnel: w668 -> [w676 w681 w687 w692]
            tunnel: w667 -> [w675 w680 w685 w691]
            tunnel: w665 -> [_ _ _ w690]
            frame 0, Default {
              n255 = call "laserOnOff.vi"("error in (no error)"=w676, "Emission (F = OFF)"=w675, "VISA Refnum in"=w677) -> ("error out"=w679:errorcluster, "VISA Refnum out"=w678:refnum<visa-resource-name>)  [unwired: 6 in, 1 out]
              n256 = local write "406 Emission"(w675) -> ()
            }
            frame 1 {
              n257 = call "laserOnOff.vi"("error in (no error)"=w681, "Emission (F = OFF)"=w680, "VISA Refnum in"=w682) -> ("error out"=w684:errorcluster, "VISA Refnum out"=w683:refnum<visa-resource-name>)  [unwired: 6 in, 1 out]
              n258 = local write "532 Emission"(w680) -> ()
            }
            frame 2 {
              n259 = call "laserOnOff.vi"("error in (no error)"=w687, "Emission (F = OFF)"=w685, "VISA Refnum in"=w686) -> ("error out"=w689:errorcluster, "VISA Refnum out"=w688:refnum<visa-resource-name>)  [unwired: 6 in, 1 out]
              n260 = local write "662 Emission"(w685) -> ()
            }
            frame 3 {
              n261 = call "laserOnOff.vi"("error in (no error)"=w692, "Emission (F = OFF)"=w691, "VISA Refnum in"=w690) -> ("error out"=w694:errorcluster, "VISA Refnum out"=w693:refnum<visa-resource-name>)  [unwired: 6 in, 1 out]
              n262 = local write "785 Emission"(w691) -> ()
              n263 = local write "All Emit"(w691) -> ()
            }
          }
          n264 = VISA Close(VISA resource name=w673, error in (no error)=w674) -> (error out=w666:errorcluster)
        }
        n265 = local write "Status"("" ("Status")) -> ()
        n266 = VISA Close(VISA resource name=w660, error in (no error)=w652) -> (error out=w653:errorcluster)
      }
    }
    n267 = case shown="True" "Auto Filter" {
      tunnel: [w363 w365] -> w347
      tunnel: w346 -> [w363 w364]
      frame False {
      }
      frame True {
        # "This is the timer for the filtering routine."
        n268 = call "Elapsed Time"("Time Target (s)"="Time Target (s)", "Auto Reset"=TRUE, "error in (no error)"=w364) -> ("Elapsed Time (s)"=w368:dbl, "Time has Elapsed"=w370:bool, "error out"=w369:errorcluster)  [unwired: 9 in, 5 out]
        "Time has Elapsed" <- w370
        n269 = Divide(x=w368, y=60.0) -> (x/y=→"Elapsed Time (min)":dbl)
        n270 = property on="Time has Elapsed" class="Bool (strict)"(error in=w369, "Val(Sgnl)"=w370) -> (error out=w365:errorcluster)  [unwired: 1 in, 1 out]
      }
    }
  }
  n271 = Unbundle By Name("Acquisition Settings") -> ("Down Sample Ratio"=w1:u32)
  n272 = call "picoGetTimebase.vi"("error in (no error)"=w11, "Rapid Block Acquisition Settings"="Acquisition Settings", "handle in"=w8) -> ("error out"=w10:errorcluster, "Sample Interval"=w5:sgl, "handle out"=w9:i16)  [unwired: 6 in]
  n273 = call "picoTrigger.vi"("Trigger Channel Settings"="Channel B Settings", "error in (no error)"=w10, "maxADC"=w6, "Trigger Settings"="Trigger Settings", "Handle In"=w9) -> ("error out"=w18:errorcluster, "Range"=w15:u16, "handle out"=w17:i16)  [unwired: 4 in]
  n274 = call "picoSetMem.vi"("error in (no error)"=w18, "Rapid Block Acquisition Settings"="Acquisition Settings", "Handle In"=w17) -> ("error out"=w3:errorcluster, "timebase"=w20:u32, "postTriggerSamples"=w21:u32, "Handle Out"=w22:i16, "nCaptures"=w19:u16)  [unwired: 4 in]
  n275 = call "picoExtractSettings.vi"("Rapid Block Acquisition Settings"="Acquisition Settings") -> ("Down-Sample Mode"=w12:i32, "Down Sample Ratio"=w13:u32, "Numeric"=w14:i32)  [unwired: 8 in]
  n276 = while {
    tunnel: [w726] -> w23
    tunnel: w22 -> [w725]
    tunnel: w21 -> [w724]
    tunnel: w20 -> [w723]
    tunnel: w19 -> [w730]
    tunnel: w6 -> [w716]
    tunnel: w15 -> [w717]
    tunnel: w14 -> [w720]
    tunnel: w13 -> [w715]
    tunnel: w12 -> [w714]
    tunnel: w5 -> [w709]
    tunnel: w3 -> [w703]
    tunnel: w1 -> [w697]
    stop <- w712 stop-if-true
    n277 = call "picoRunBlock.vi"("error in (no error)"=w703, "timebase"=w723, "postTriggerSamples"=w724, "Handle In"=w725) -> ("error out"=w729:errorcluster, "handle"=w728:i16)  [unwired: 5 in, 1 out]
    n278 = call "picoReady.vi"("error in (no error)"=w729, "handle in"=w728) -> ("error out"=w727:errorcluster, "handle out"=w722:i16)  [unwired: 8 in]
    n279 = Wait Until Next ms Multiple(millisecond multiple=u32 1000 ("milliseconds to wait")) -> ()  [unwired: 1 out]
    n280 = Multiply(x=w709, y=w697) -> (x*y=w705:sgl)
    n281 = call "picoGetValues.vi"("Down-Sample Mode"=w714, "Down Sample Ratio"=w715, "nCaptures"=w730, "error in (no error)"=w727, "postTriggerSamples"=w720, "Handle In"=w722) -> ("error out"=w719:errorcluster, "buffer"=w707:i16[][], "handle"=w726:i16)  [unwired: 3 in]
    n282 = call "picoCoAdd.vi"("error in (no error)"=w719, "Buffer In"=w707) -> ("error out"=w718:errorcluster, "Waveform Out"=w708:dbl[])  [unwired: 8 in]
    n283 = call "picoToVolts.vi"("error in (no error)"=w718, "Max_adc"=w716, "Range Index"=w717, "Data"=w708) -> ("error out"=w701:errorcluster, "Data (mV)"=w704:dbl[])  [unwired: 6 in]
    n284 = local read "PAS Save"() -> (w696:bool)
    n285 = local read "crd"() -> (w698:path)
    n286 = Bundle(0, w705, "Data (mV)"=w704) -> (→"Channel A":cluster{i32, sgl, "Data (mV)":dbl[]})  [unwired: 1 in]
    n287 = call "Get Tau.vi"("CalType"=analys_meth."LRS", "Dt"=w705, "X"=w704) -> ("tau"=w702:dbl)  [unwired: 5 in, 3 out]
    "tau" <- w702
    n288 = call "saveTimeSeries_IV.vi"("1"=w702, "file path (dialog if empty)"=w698, "save?"=w696, "Error In"=w701, "Number of Data Series"=enum16{"1", "2", "3", "4"}."1") -> ("Error Out"=w700:errorcluster)  [unwired: 10 in]
    n289 = local read "Exit"() -> (w695:bool)
    n290 = Unbundle By Name(w700) -> ("status"=w711:bool)
    n291 = Or(x=w711, y=w695) -> (x .or. y?=w712:bool)
  }
  n292 = call "PicoScope2000aClose.vi"("handle"=w23) -> ()  [unwired: 11 in]
  n293 = Release Queue(queue=w36, error in (no error)=w35) -> ()  [unwired: 1 in, 3 out]
  n294 = Merge Errors(w85, w76) -> (w84:errorcluster)
  n295 = Release Queue(queue=w33, error in (no error)=w32) -> ()  [unwired: 1 in, 3 out]
  n296 = call <vilib>:"Simple Error Handler.vi"("error in (no error)"=w84) -> ("error out"=w83:errorcluster)  [unwired: 4 in, 4 out]
  n297 = flat-sequence {
    tunnel: w83 -> [w731]
    tunnel: [w731] -> w82
    frame #0 {
      n298 = local write "Exit"(FALSE) -> ()
    }
  }
  "Error Console" <- w82
